vi "ChangeOverGui.vi"() -> ()   [LabVIEW 2016]
uses:
  ChangeOverGui.Properties.ctl
  Logger/Logger.Variant.Sets.ctl
  Station/Station.Changeover.State.vi
  Station/Station.Plate.Properties.ctl
  Sequence/Sequence.Code.SerialFormat.ctl
  Drivers/V7310/LowLevel/V7310.Job.Sets.ctl
  ChangeOverGui.Action.ctl
  Station/Station.State.ctl
  Sequence/Sequence.MainMode.ctl
  Sequence/Sequence.PlateType.ctl
  <vilib>/Utility/miscctls.llb/LVBoundsTypeDef.ctl
  <vilib>/Utility/miscctls.llb/LVRowAndColumnUnsignedTypeDef.ctl
  tools/CitTemplate/citTemplate.errData.ctl
  tools/EventLog/EventLog.EventSource.ctl
  tools/Translator/Translator.Message.ctl
  tools/Config/Config.Global.vi
  Global/ApplicationGlobal.vi
  Station/Station.Global.vi
  Sequence/Sequence.Global.vi
  Drivers/V7310/LowLevel/V7310.Global.vi
  tools/Picture/Rotate.llb/rotate 24bit.vi
panel:
  out "Progress":bool
  out "TotalCounter":u32 caption="Total Counter"
  in  "ShowOrdersTable":bool
  in  "OrdersTable":i32(listbox) caption="Last A"
  in  "ShowPropertiesClient":bool
  out "DoubleOrder":bool
  in  "ShowPropertiesWabco":bool
  in  "Properties":T1={"LaserJob"=0, "AddTxt"="", "FactoryCode"="", "RevID"=0, "ForkID"=0, "Failures Limit"=0, "GlobalCounter"=0, "Bank"=enum."A/B-1", "SerialFormat"=enum."6 dig", "CodeA"={"X"=0.0, "Y"=0.0, "Angle"=0.0}, "CodeB"={"X"=0.0, "Y"=0.0, "Angle"=0.0}, "SetupDMC"=FALSE, "CVX Program"=0} {"CodeB"."Angle" format="%.1f"; "CodeB"."Y" format="%.2f"; "CodeB"."X" format="%.2f"; "CodeA"."Angle" format="%.1f"; "CodeA"."Y" format="%.2f"; "CodeA"."X" format="%.2f"; "LaserJob" items=["", "000 000 000 0", "899 010 203 4", "899 010 206 4", "899 050 124 4", "899 050 145 4", "899 050 146 4", "899 050 146 4v bst3", "899 050 147 4", "899 052 580 4", "899 052 580 4v2", "899 052 582 4", "899 052 930 4", "899 052 942 4", "899 052 942 4 v2", "899 053 089 4", "899 053 089 4v 9325100100", "899 053 096 4", "899 053 096 4 v2", "899 053 502 4", "899 053 522 4", "899 053 524 4", "899 053 527 4", "899 053 803 4 v1", "899 053 803 4 v2", "899 053 803 4 v3", "899 053 803 4 v5 cb1", "899 053 804 4", "899 053 804 4 V2", "899 053 804 4 v 4324101170", "899 053 804 4 v daiml", "899 053 804 4_scania", "899 053 804 4v daimler", "899 053 804 4v daimler2", "899 053 804 4v047", "899 053 814 4", "899 053 814 4 v1", "899 053 814 4_KESKA", "899 053 814 4v sc", "899 053 815 4 ", "899 053 913 4", "899 053 913 4 test", "899 053 913 4 v2", "899 053 923 4", "8990501244", "Karol 899 053 089 4", "VJ Test", "inne"]}
  in  "ViewMode":enum16{"-", "Wabco", "Client"}(ring)
  in  "Serial":T2
  in  "Wabco":cluster{"ProductNo":string, "PlateNo":string}
  in  "Client":cluster{"ProductNo":string, "PlateNo":string}
  out "ClientPlate":picture
  out "Image":picture
  out "WabcoPlate":picture
  out "_loop":i32(ring)=4
  out "Panel":refnum<vi>
  in  "StartHere...":bool
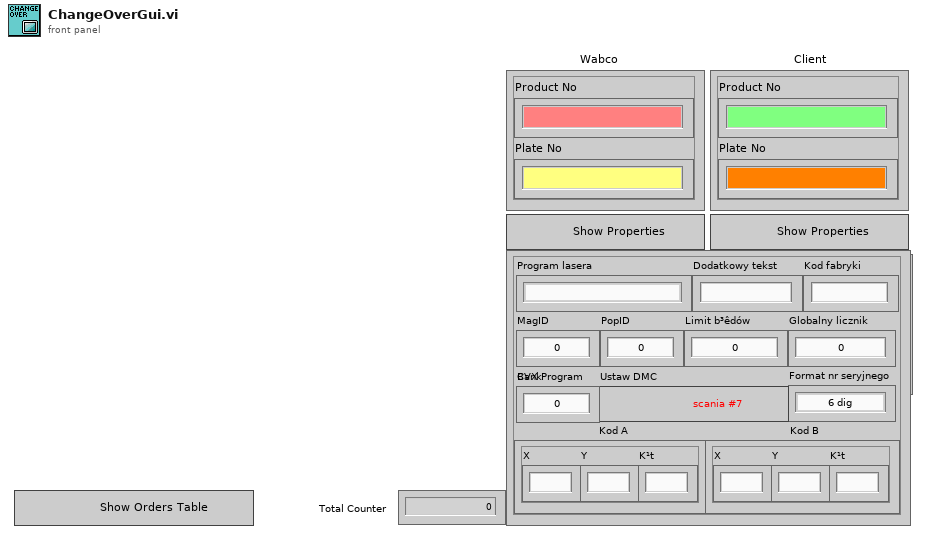
[diagram p1: front panel]
types:
  T1 = typedef "ChangeOverGui.Properties.ctl" = cluster{"LaserJob":u16, "AddTxt":string, "FactoryCode":string, "RevID":u8, "ForkID":u8, "Failures Limit":u16, "GlobalCounter":i32, "Bank":enum8{"A/B-1", "A/B-2", "A/B-3"}, "SerialFormat":enum16{"", "6 dig", "7 dig"}, "CodeA":cluster{"X":dbl, "Y":dbl, "Angle":dbl}, "CodeB":cluster{"X":dbl, "Y":dbl, "Angle":dbl}, "SetupDMC":bool, "CVX Program":u8}
  T2 = cluster{"TotalQuantity":u16, "OrderQuantity":u16, "SerialNo":i32}
  T3 = typedef "Logger.Variant.Sets.ctl" = cluster{"State":T4, "ImgPath":path, "WabcoPlate":string, "WabcoProduct":string, "ClientProduct":string, "ClientPlate":string, "TotalQuantity":u16, "OrderQuantity":u16, "Serial":i32, "Wabco":T5, "Client":T5}
  T4 = typedef "Station.Changeover.State.vi" = enum16{"Init", "Scaning", "NOK", "Wait for ack", "Ready"}
  T5 = typedef "Station.Plate.Properties.ctl" = cluster{"LaserJob":string, "AdditionalTxt":string, "FactoryCode":string, "RevID":u8, "ForkID":u8, "FailuresLimit":u16, "GlobalCnt":i32, "ScannerProgram":u8, "SerialFormat":T6, "CoordA":T7, "CoordB":T7, "DMCconfig":i32, "CVX_Program":u16}
  T6 = typedef "Sequence.Code.SerialFormat.ctl" = enum8{"", "6 dig", "7 dig"}
  T7 = typedef "V7310.Job.Sets.ctl" = cluster{"X":dbl, "Y":dbl, "Angle":dbl}
  T8 = typedef "Station.State.ctl" = enum16{"Idle", "Ready", "Run", "Stop", "Error", "Home", "Done", "Emg"}
  T9 = typedef "ChangeOverGui.Action.ctl" = enum32{"idle", "constructor", "destructor", "---ChangeOverGui ---", "Clear", "Validate", "Read File", "Read Imgs", "Check", "Accept", "Reject", "Scan.Begin", "Scan", "Update Table", "Update Counter", "DMC Accept"}
  T10 = typedef "Sequence.MainMode.ctl" = enum16{"Process", "Base", "Order", "Manual", "Logs", "Results", "Stats", "DMC Config"}
  T11 = typedef "Sequence.PlateType.ctl" = enum16{"Wabco", "Client"}
  T12 = typedef "LVRowAndColumnUnsignedTypeDef.ctl" = cluster{"Row":u32, "Column":u32}
  T13 = typedef "citTemplate.errData.ctl" = cluster{"ts":timestamp, "src":T14, "instance":i32, "action":string, "error":errorcluster, "unconfirmed":bool}
  T14 = typedef "EventLog.EventSource.ctl" = enum16{"All", "Gui", "Ref", "File", "Arch", "Seq", "CPX", "DB", "Laser", "Scan.P", "Scan.O"}
  T15 = enum8{"Enabled", "Disabled", "Disabled and Grayed Out"}
  T16 = typedef "Translator.Message.ctl" = enum16{"-", "Event confirmed", "Log out", "Log in", "Shutdown", "Cancel", "Start", "Begin time", "End time", "Duration", "Service Mode", "Ignore Results", "Serial Format", "On", "Off", "OK", "NOK", "NOK %s", "Home", "Work", "Close", "Open", "In progress...", "Missing", "Empty", "Hardware failure", "Initial", "Default", "Total", "Out of range", "Free disk space is below 1GB - contact technician", "Error %d >> %s", "Error %d >> %s >> %s", "Msg %d >> %s", "Laser msg %d %s", "Laser cmd error %s %d", "Laser cmd failed %s", "Laser cmd warning %s", "Laser disconnected", "Laser status %s", "Laser already started", "Laser job unkonwn %s", "Laser job missing %s", "Laser job select failure %s", "Unable to start laser printing (%s)", "Unable to stop laser printing (%s)", "Laser marking aborted", "Laser marking timeout", "Unable to reset Laser Interlock (%s)", "Unable to trigger Laser. Laser not ready (%s)", "Laser job '%s' coordinates not configured", "Starting %s", "Quitting %s", "Configured", "Initializing", "Quitting", "Loading", "Loaded %d results", "Loaded %d events", "Running", "Stopped", "Summary", "Laser", "Do you want to continue?", "Do you want to delete the configuration?", "The configuration is being used by an order. Unable to delete!", "Press confirm button", "Station is not based. Do you want to exit?", "Station requires changeover. Do you want to run the test?", "Test options are not set as default. Do you want to continue?", "Formatting of WabcoNo is disabled. Do you want to continue?", "Product not detected. Do you want to continue?", "Product scan failed. Do you want to continue?", "Calibration", "Log out?", "System", "All", "IDLE", "Translating...%s", "Not found", "Alarm %s", "Run", "Skip", "Abort", "Repeat", "Please wait...", "Database disconnected", "Database disconnected - changeover disabled!", "Login to database successful", "Login to database failed: %d; %s", "Unable to check the product status of reference %d - database disconnected", "Unable to set the product status of reference %d - database disconnected", "Variant file backup %s", "Read variant (%s)", "Result", "Station armed!", "Station requires changeover!", "Select reference number...", "EMERGENCY BUTTON - press Control button", "EMERGENCY DOOR - press Control button", "Resetting Emergency...", "Unable to reset safety circuit - Emergency Button pressed", "Unable to reset safety circuit - Emergency Side Door open", "Station not based", "Station based", "Station not empty", "Station basing...", "No order", "Press Start to begin new order", "Scanning new order", "Order NOK. Correct or scan again", "Order OK. Press Accept", "Order ready", "Revolver incorrect", "Fork incorrect", "Revolver missing", "Revolver empty", "Container missing", "Offline results", "Offline statistics", "Updating statistics %.1f %%", "DMC Configurator", "Door open", "Close the front door", "Press start button", "Done. Open the front door", "Running...", "Running...%.1f %%", "Pause %s", "Pause %s. NOK container missing", "Pause %s. OK container missing", "Pause %s. Revolver empty", "Pause %s. Revolver missing", "Pause %s. Revolver incorrect", "Pause %s. Fork missing", "Pause %s. Fork incorrect", "Pause %s. Too many failures", "Pause %s. Unloading failure", "Pause %s. One slot is not working", "Pause %s. Part order is done. Empty OK container", "Pause %s. Unable to move product to slot", "Pause %s. Unable to move back product pusher", "Pause %s. Unable to lift product", "Pause %s. Unable to move back product lifter", "Pause %s. Unable to move product arm to Work", "Pause %s. Unable to move product arm to NOK", "Pause %s. Unable to move product arm to OK", "Pause %s. Unable to unsuck the NOK product", "Pause %s. Unable to drop the NOK product", "Pause %s. Product OK missing", "Pause %s. Unable to unsuck the OK product", "Pause %s. Unable to drop the OK product", "Stopping...", "File '%s' is missing", "File '%s' is broken", "File '%s' is running", "Log file started (%s)", "Log file ended (%s)", "Log file stopped (%s)", "Log file ignored (%s)", "Log file exported (%s)", "Log file export failed (%s)", "Wrong serial number in log file", "Wrong reference number in log file", "Test steps are missing", "%s = %.3f", "Process param '%s' not found in DB", "Process param '%s' wrong order", "Process param '%s' value %.3f out of limits (%.3f; %.3f)", "Step%d param '%s' not found in DB", "Step%d param '%s' wrong order", "Step%d param '%s' value %.3f out of limits (%.3f; %.3f)", "Step%d EV '%s' not found in DB", "Step%d EV '%s' wrong order", "\"%s\" not found in DB", "\"%s\" wrong order", "\"%s\" value %.3f out of limits (%.3f; %.3f)", "\"%s\" not found in software", "Process init (%s)", "Process started", "Process restarted", "Process run", "Process done", "Process done - remove OK container", "Process aborted", "Process aborted at work", "Process aborted at home", "Process error", "Process error at home", "Process error at work", "Process close", "Process pause", "Process continue", "Process door open", "Process door close", "Process pause at slot %s due to %s", "Select plate from the order to process", "Do you want to start the process?", "Do you want to continue the process?", "There is unfinished order. Do you want to put the new order?", "Product %s %d OK", "Product %s %d NOK", "Unable to unload the slot %s. Product missing in the slot", "Unable to unload the slot %s. Product already in the arm", "Unable to accept the product as OK. Product missing in slot %s", "Unable to accept the product as OK. Product could not drop into the container at slot %s", "Unable to accept the product as NOK. Product could not drop into the container at slot %s", "Scan failed. Error %s", "Scan failed. Scanner disconnected", "Scan failed. Wrong Wabco number %d, limit (%d,%d)", "Scan failed. Wrong serial number %d, limit (%d,%d)", "Scan failed. Wrong date %d, limit (%d,%d)", "Scan failed. Wrong product wabco number %d (expected %d)", "Scan failed. Wrong product serial number %d (expected > 0)", "Scan OK %s", "Scan failed. Unable to determine table position (%s)", "Scan failed. Timeout", "Tune failed. Scanner disconnected", "Tune failed. Timeout", "%s = %d", "%s = %d->%d", "Unable to set %s = %.2f - Air Pressure Inside off", "Unable to set digital output '%s' = %d", "Unable to activate air pressure inside - timeout", "Unable to activate air pressure inside - aborted", "Unable to switch on Air Main Valve - Air Pressure Inlet off", "Unable to switch on Air Main Valve - Door open", "Unable to switch off Air Main Valve - timeout", "Unable to switch off Air Main Valve - aborted", "Unable to rotate Table - timeout", "Unable to rotate Table - aborted", "Unable to rotate Table - Product Move not in Home position", "Unable to rotate Table - Air Pressure Inside off", "Unable to rotate Table - Product Lift A not in Home position", "Unable to rotate Table - Product Lift B not in Home position", "Unable to rotate Table - unlock before movement timeout", "Unable to rotate Table - lock after movement timeout", "Unable to move Table Lock to %s position - timeout", "Unable to move Table Lock to %s position - aborted", "Unable to move Table Lock to %s position - Air Pressure Inside off", "Unable to move Table Lock to %s position - Table not in position", "Unable to move Product Lift A to %s position - timeout", "Unable to move Product Lift B to %s position - timeout", "Unable to move Product Lift A to %s position - aborted", "Unable to move Product Lift B to %s position - aborted", "Unable to move Product Lift A to %s position - Air Pressure Inside off", "Unable to move Product Lift B to %s position - Air Pressure Inside off", "Unable to move Product Lift A to %s position - Table not locked", "Unable to move Product Lift B to %s position - Table not locked", "Unable to move Product Lift A to %s position - Product Arm not in Work position", "Unable to move Product Lift B to %s position - Product Arm not in Work position", "Unable to set Product Suction Gripper %s to %s - timeout", "Unable to set Product Suction Gripper %s to %s - aborted", "Unable to set Product Suction Gripper %s to %s - Air Pressure Inside off", "Unable to set Product Suction Gripper %s to %s - Table slot unkown", "Unable to move Product Arm to %s position - timeout", "Unable to move Product Arm to %s position - aborted", "Unable to move Product Arm to %s position - Air Pressure Inside off", "Unable to move Product Arm to %s position - Product Lift A not in Home position", "Unable to move Product Arm to %s position - Product Lift B not in Home position", "Unable to move Product to %s position - timeout", "Unable to move Product to %s position - aborted", "Unable to move Product to %s position - Air Pressure Inside off", "Unable to move Product to %s position - Table not in position"}
  T17 = typedef "citTemplate.notifierHandle.ctl" = refnum<notifier>
  T18 = enum32{"Invalid", "Standard", "Closed", "Hidden", "Minimized", "Maximized"}
  T19 = typedef "Station.Data.ctl" = cluster{"State":T8, "Seq.State":T20, "Seq.BreakReason":T21, "Seq.BreakSource":T22, "Hw failure":bool, "Unconfirmed":bool, "Station empty":bool, "Home err":bool, "Order done":bool, "DUT present":T23, "EmgState":T24, "Sets":T25, "StatusBits":T27}
  T20 = typedef "Sequence.State.ctl" = enum16{"Init", "Idle", "Home", "Work", "Run", "Pause"}
  T21 = typedef "Sequence.Test.BreakReason.ctl" = enum16{"-", "NOK container", "OK container", "Rev empty", "Rev missing", "Rev wrong", "Fork missing", "Fork wrong", "NOK limit", "Unload failure", "Single slot", "Part done", "Err: Prod move work", "Err: Prod move home", "Err: Prod lift work", "Err: Prod lift home", "Err: Prod Arm Work", "Err: Prod Arm NOK", "Err: Prod Arm OK", "Err: Prod NOK suck", "Err: Prod NOK drop", "Err: Prod OK missing", "Err: Prod OK suck", "Err: Prod OK drop"}
  T22 = typedef "Sequence.Test.BreakSource.ctl" = enum16{"-", "A", "B", "A/B"}
  T23 = typedef "FestoCPX.Station.ProdPresent.ctl" = cluster{"Slot1":cluster{"A":bool, "B":bool}, "Slot2":cluster{"A":bool, "B":bool}, "Slot3":cluster{"A":bool, "B":bool}, "Slot4":cluster{"A":bool, "B":bool}, "Final":cluster{"A":bool, "B":bool}, "OK":cluster{"A":bool, "B":bool}, "Container":cluster{"OK":bool, "NOK":bool}}
  T24 = typedef "FestoCPX.Station.EmgState.ctl" = cluster{"Button":bool, "SideDoor":bool, "FrontDoor":bool, "DoorSecured":bool}
  T25 = typedef "Sequence.UserData.ctl" = cluster{"GuiMode":T10, "Test":T26, "ContinueOrder":bool}
  T26 = typedef "MainGui.TestOptions.ctl" = cluster{"IgnoreResults":bool, "IgnoreImages":bool, "ServiceMode":bool}
  T27 = typedef "Station.Home.Status.Bits.ctl" = cluster{"Door Close":bool, "Rev OK":bool, "Fork OK":bool, "Container OK":bool, "Station empty":bool}
  T28 = typedef "LVBoundsTypeDef.ctl" = cluster{"Width":u32, "Height":u32}
  T29 = typedef "LVPositionTypeDef.ctl" = cluster{"Left":i32, "Top":i32}
  T30 = typedef "Sequence.Data.ctl" = cluster{"BeginTS":timestamp, "EndTS":timestamp, "State":T20, "Status.Work":T31, "Status.Process":T31, "Status.Home":T31, "Status.Wabco":T31, "Status.Client":T31, "BreakReason":T21, "BreakSource":T22, "DoorLock":bool, "Status.Prod":T32[], "UserAction":T36, "UserData":T25, "Error":errorcluster, "Code":T37, "Rotations":i32, "ProdIdx":i32, "ProdDone":T32[], "PrintedSerials-Wabco":i32[], "PrintedSerials-Client":i32[], "Counters-Wabco":T38, "Counters-Client":T38}
  T31 = typedef "Sequence.Step.Status.ctl" = enum16{"-", "Pending", "Running", "Skipped", "Passed", "Failed", "Done", "Error", "Aborted", "Stopped"}
  T32 = typedef "Sequence.Test.Status.ctl" = cluster{"Slot":T33, "A":T35, "B":T35}
  T33 = typedef "Sequence.Slot.StatusData.ctl" = cluster{"ID":i32, "Unload":T34, "TS":timestamp, "duration":u32}
  T34 = typedef "Sequence.Test.Unload.Status.ctl" = enum16{"init", "check NOK", "check OK", "wait on NOK", "wait on OK", "wait on Unload", "done"}
  T35 = typedef "Sequence.Prod.StatusData.ctl" = cluster{"status":T31, "pause":T21, "present":bool, "printed":bool, "scanned":bool, "tuned":bool, "removed":bool, "OCRignored":bool, "LaserVariables":string[], "Serial":i32, "path":path, "corners":cluster{"X":i32, "Y":i32}[], "verification":u8, "ScanerReadOut":string[]}
  T36 = typedef "Sequence.UserActions.ctl" = cluster{"Stop":bool, "Pause":bool, "Next":bool}
  T37 = typedef "Sequence.Code.Sets.ctl" = cluster{"Ready":bool, "DoubleOrder":bool, "OrderDone":bool, "AllowSingleSlot":bool, "IgnoreOCR":bool, "ThresholdA":u8, "ThresholdB":u8, "Plate":T11, "ImgPath":path, "Variant":T3}
  T38 = typedef "Sequence.Counters.ctl" = cluster{"Expected":u16, "Done":u16, "OK":u16, "NOK":u16, "NOKlimit":u16, "Part":u16, "PartOK":u16}
  T39 = typedef "V7310.Data.Status.ctl" = cluster{"State":T40, "LaserStatus":T41, "LaserStatusRaw":string, "Ref":refnum<k5>, "RTC TS":timestamp, "Conn TS":timestamp, "Msg":T42[], "JobInUse":string, "Jobs":string[], "Vars":T43[]}
  T40 = typedef "V7310.Data.Status.State.ctl" = enum16{"First", "Init", "Msg", "Error", "Abort", "Idle", "Run"}
  T41 = typedef "V7310.LaserStatus.ctl" = enum16{"-", "FatalError", "Initialize", "KeySwitchOpen", "TimeoutInterlock", "InterlockOpen", "StartUp", "ShutterlockOpen", "Standby", "Ready", "PrepareForMarking", "WaitForTrigger", "Marking"}
  T42 = typedef "V7310.Message.Data.ctl" = cluster{"ID":i32, "Msg":string}
  T43 = typedef "V7310.Job.Variable.ctl" = cluster{"Name":string, "Value":string}
  T44 = typedef "DMCConfiguatorGui.ConfigData.ctl" = cluster{"CreateDate":timestamp, "Name":string, "Components":T45[]}
  T45 = typedef "DMCConfiguatorGui.Component.ctl" = cluster{"Type":T46, "Var":T47, "Text":string}
  T46 = typedef "DMCConfiguatorGui.Type.ctl" = enum8{"Text", "Variable"}
  T47 = typedef "DMCConfiguatorGui.Var.ctl" = enum8{"-", "Wabco No", "Client No", "Serial", "Date"}
  T48 = typedef "imagedata.ctl" = cluster{"image type":i32, "image depth":i32, "image":u8[], "mask":u8[], "colors":u32[], "Rectangle":cluster{"left":i16, "top":i16, "right":i16, "bottom":i16}}
  T49 = cluster{"WabcoProduct":string, "WabcoPlate":string}
  T50 = cluster{"ClientProduct":string, "ClientPlate":string}
  T51 = cluster{"TotalQuantity":u16, "OrderQuantity":u16, "Serial":i32}
  T52 = typedef "Keyence.CodeDetails.ctl" = cluster{"text":string, "status":bool, "corners":cluster{"X":i32, "Y":i32}[], "level":u8, "class":string, "path":path}
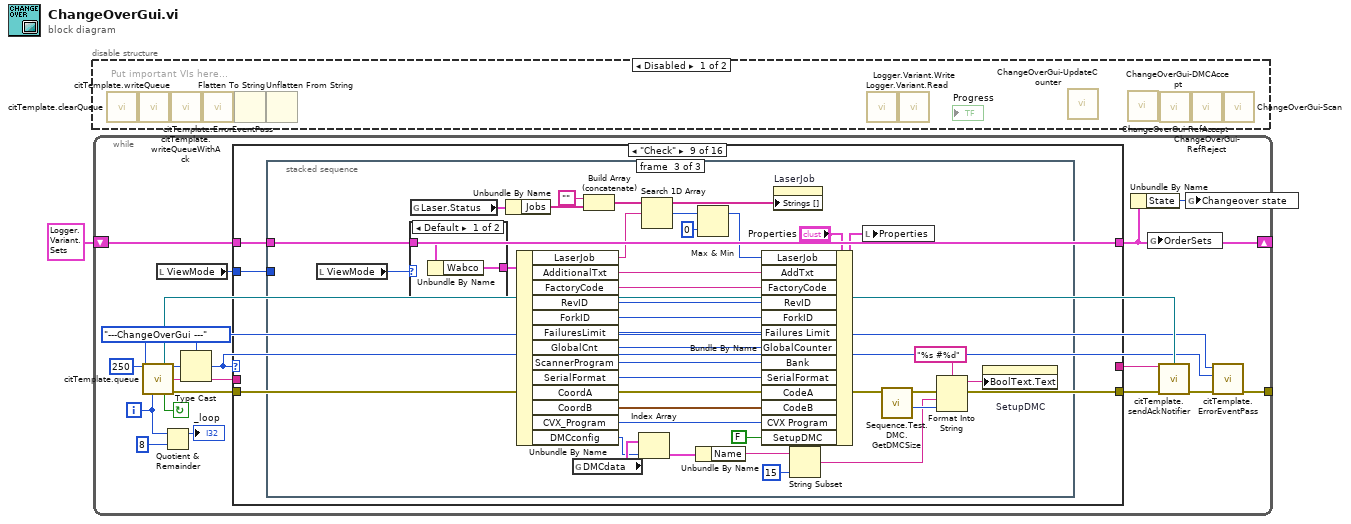
[diagram p0: block diagram]
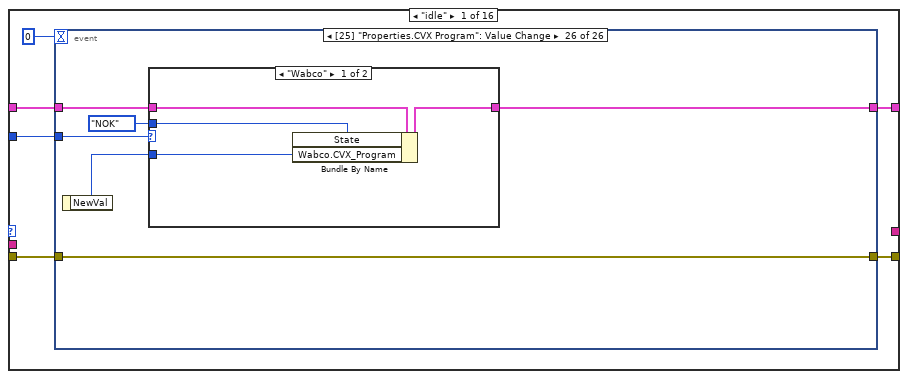
[diagram p3: hidden frame]
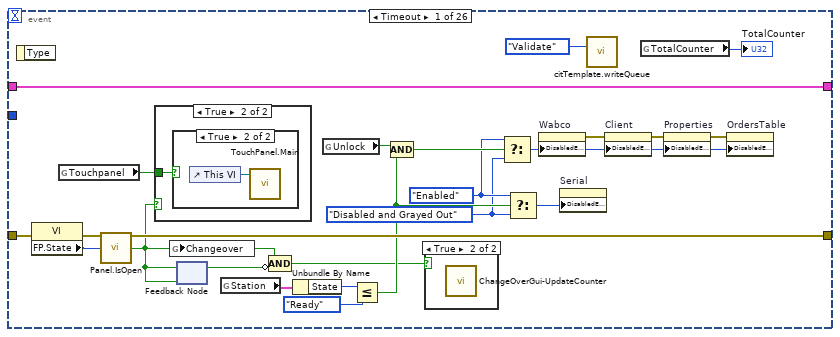
[diagram p4: hidden frame]
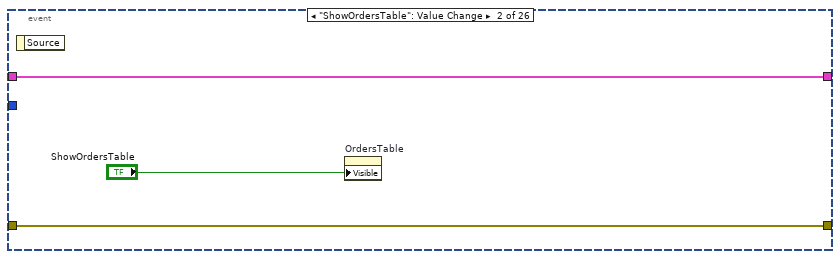
[diagram p8: hidden frame]
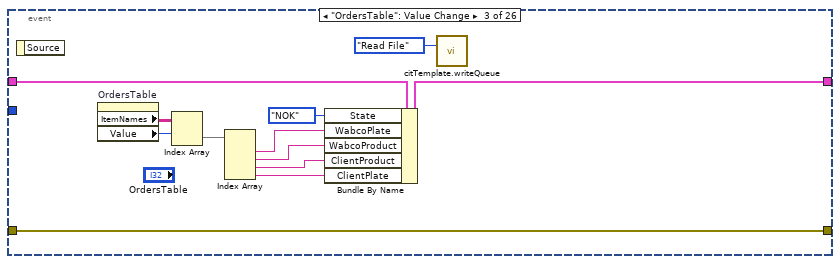
[diagram p9: hidden frame]
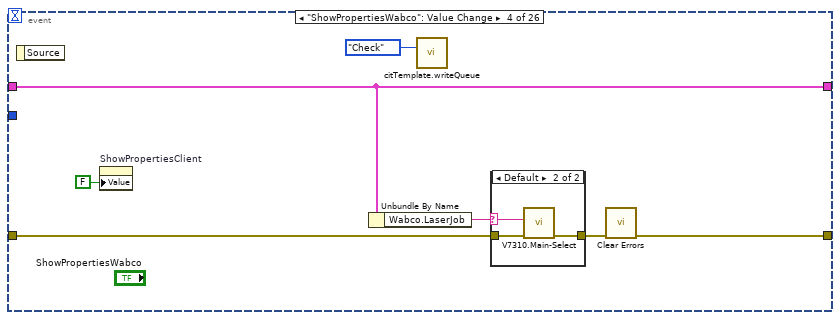
[diagram p10: hidden frame]
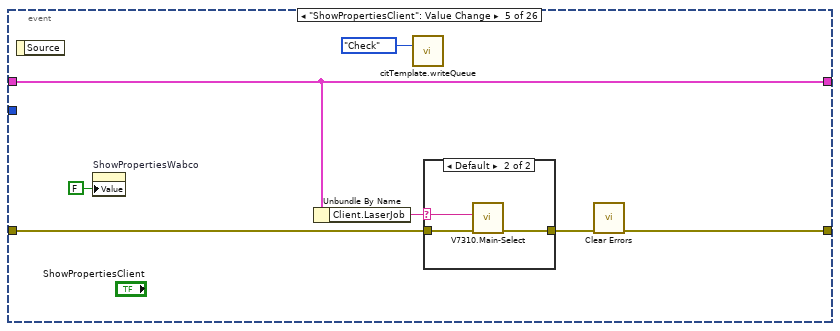
[diagram p12: hidden frame]
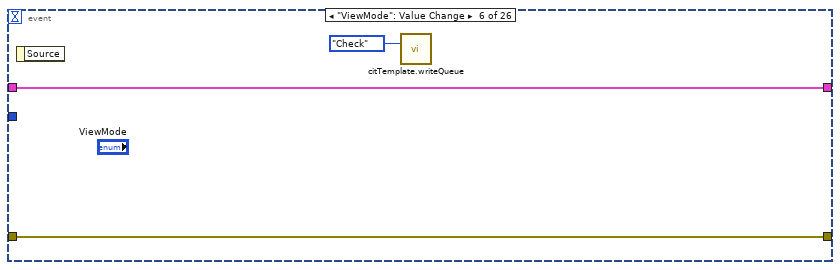
[diagram p14: hidden frame]
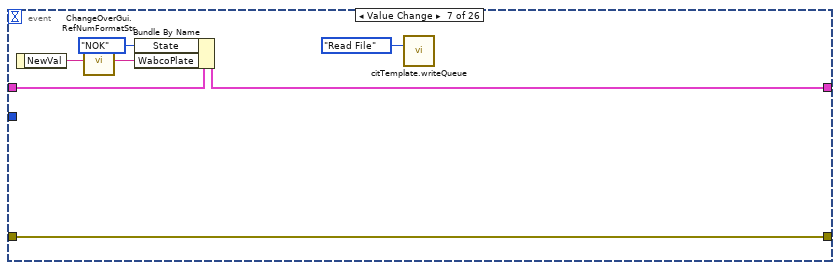
[diagram p15: hidden frame]
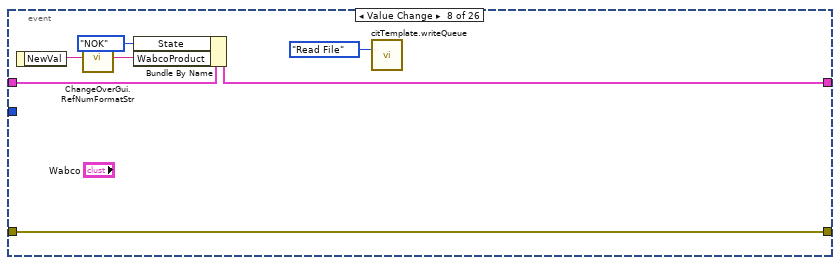
[diagram p16: hidden frame]
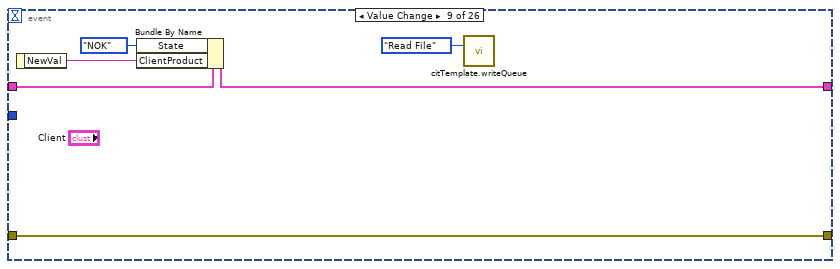
[diagram p17: hidden frame]
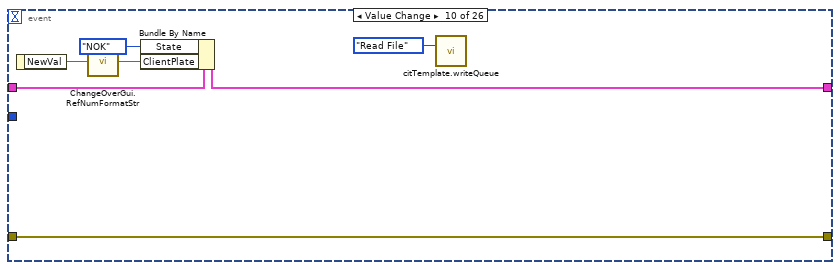
[diagram p18: hidden frame]
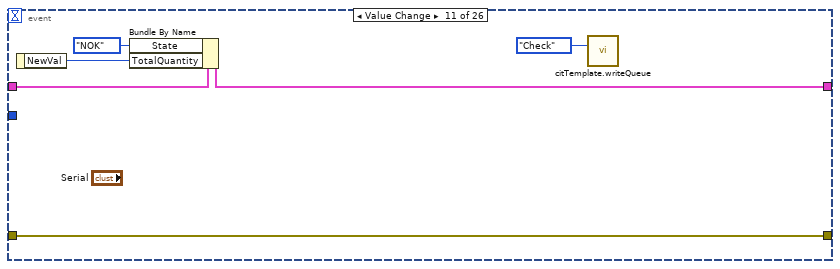
[diagram p19: hidden frame]
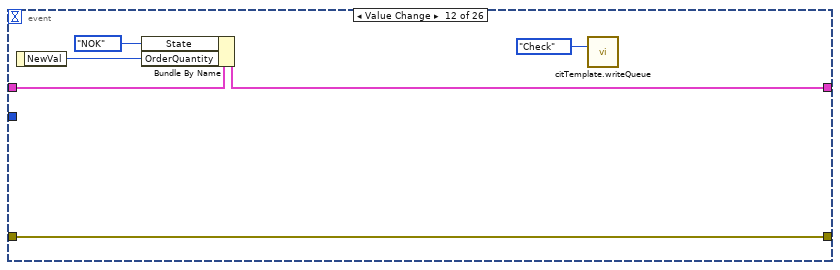
[diagram p20: hidden frame]
diagram:
  n1 = disable-structure shown="Disabled" {
    frame Disabled {
      # "Put important VIs here..."
      n2 = call "citTemplate.clearQueue.vi"() -> ()  [unwired: 14 in, 2 out]
      n3 = call "citTemplate.writeQueue.vi"() -> ()  [unwired: 15 in, 1 out]
      n4 = call "citTemplate.writeQueueWithAck.vi"() -> ()  [unwired: 13 in, 3 out]
      n5 = call "citTemplate.ErrorEventPass.vi"() -> ()  [unwired: 11 in, 1 out]
      n6 = Flatten To String() -> ()  [unwired: 4 in, 3 out]
      n7 = Unflatten From String() -> ()  [unwired: 5 in, 3 out]
      n8 = call "Logger.Variant.Read.vi"() -> ()  [unwired: 6 in, 6 out]
      n9 = call "Logger.Variant.Write.vi"() -> ()  [unwired: 11 in, 1 out]
      n10 = call "ChangeOverGui-UpdateCounter.vi"() -> ()  [unwired: 11 in, 1 out]
      n11 = call "ChangeOverGui-DMCAccept.vi"() -> ()  [unwired: 11 in, 1 out]
      n12 = call "ChangeOverGui-RefAccept.vi"() -> ()  [unwired: 11 in, 1 out]
      n13 = call "ChangeOverGui-RefReject.vi"() -> ()  [unwired: 11 in, 1 out]
      n14 = call "ChangeOverGui-Scan.vi"() -> ()  [unwired: 11 in, 1 out]
    }
    frame Enabled {
    }
  }
  n15 = while {
    tunnel: [w7] -> _
    shift-right: [w2] -> _
    shift-left: T3 {"State"=enum."Init", "ImgPath"=path "", "WabcoPlate"="", "WabcoProduct"="", "ClientProduct"="", "ClientPlate"="", "TotalQuantity"=0, "OrderQuantity"=0, "Serial"=0, "Wabco"={"LaserJob"="", "AdditionalTxt"="037", "FactoryCode"="", "RevID"=0, "ForkID"=0, "FailuresLimit"=0, "GlobalCnt"=0, "ScannerProgram"=0, "SerialFormat"=enum."6 dig", "CoordA"={"X"=0.0, "Y"=0.0, "Angle"=0.0}, "CoordB"={"X"=0.0, "Y"=0.0, "Angle"=0.0}, "DMCconfig"=0, "CVX_Program"=0}, "Client"={"LaserJob"="", "AdditionalTxt"="", "FactoryCode"="037", "RevID"=0, "ForkID"=0, "FailuresLimit"=0, "GlobalCnt"=0, "ScannerProgram"=0, "SerialFormat"=enum."6 dig", "CoordA"={"X"=0.0, "Y"=0.0, "Angle"=0.0}, "CoordB"={"X"=0.0, "Y"=0.0, "Angle"=0.0}, "DMCconfig"=0, "CVX_Program"=0}} ("VariantSets out") -> [w5]
    i -> [w9]
    stop <- w16 continue-if-true
    w13 = ChangeOverGui.Action."---ChangeOverGui ---" ("Action")
    n16 = call "citTemplate.queue.vi"("ms timeout (250 ms)"=250, "event enum"=w13, "iteration (-1)"=w9) -> ("notifierHandle out"=w15:T17, "event out"=w19:u32, "(flatten) data out"=w18:string, "continue"=w16:bool, "error out"=w17:errorcluster)  [unwired: 2 in, 6 out]
    n17 = local read "ViewMode"() -> (w3:enum16{"-", "Wabco", "Client"})
    n18 = Quotient & Remainder(x=w9, y=8) -> (x-y*floor(x/y)=→"_loop":i32)  [unwired: 1 out]
    n19 = Type Cast(type=w13, x=w19) -> (*(type *) &x=w8:T9)
    n20 = case shown="\"Check\"" w8 {
      tunnel: w18 -> [_ _ _ w388 _ _ _ _ _ _ _ _ _ _ _ w1045]
      tunnel: w17 -> [w24 w334 w378 w387 w420 w428 w691 w694 w748 w825 w842 w855 w863 w1001 w1030 w1044]
      tunnel: [_ _ _ "" _ _ _ _ _ _ _ _ _ _ _ ""] -> w14
      tunnel: [w23 w333 w377 w381 w420 w428 w688 w694 w748 w824 w841 w855 w859 w1001 w1030 w1038] -> w12
      tunnel: [w21 w331 w372 w380 w421 w425 w689 w693 w747 w822 w837 w851 w865 w1002 w1029 w1037] -> w2
      tunnel: w5 -> [w22 w332 w372 w380 w421 w426 w690 w693 w747 w823 _ _ w866 w1002 w1029 w1042]
      tunnel: w3 -> [w20 _ _ _ _ w423 _ _ w746 _ _ _ _ _ w1021 w1036]
      frame "idle" {
        n21 = event shown="[25] \"Properties.CVX Program\": Value Change" {
          selector: _ -> [_ _ _ _ _ _ _ _ _ _ _ _ _ _ _ _ _ _ _ _ _ _ _ _ _ _]
          dyn-events: _ -> [_ _ _ _ _ _ _ _ _ _ _ _ _ _ _ _ _ _ _ _ _ _ _ _ _ _]
          timeout: 0 -> [_ _ _ _ _ _ _ _ _ _ _ _ _ _ _ _ _ _ _ _ _ _ _ _ _ _]
          tunnel: w24 -> [w48 w53 w65 w69 w80 w90 w95 w101 w108 w117 w123 w129 w135 w144 w161 w176 w191 w206 w221 w236 w251 w266 w281 w296 w312 w322]
          tunnel: [w46 w53 w65 w66 w77 w90 w95 w101 w108 w117 w123 w129 w135 w144 w161 w176 w191 w206 w221 w236 w251 w266 w281 w296 w314 w322] -> w23
          tunnel: w22 -> [w44 w52 w62 w70 w81 w89 w97 w104 w110 w116 w122 w128 w134 w140 w160 w174 w189 w204 w218 w233 w248 w263 w278 w293 w310 w321]
          tunnel: [w44 w52 w61 w70 w81 w89 w94 w102 w106 w115 w121 w127 w133 w139 w159 w173 w188 w203 w217 w232 w246 w262 w275 w290 w310 w317] -> w21
          tunnel: w20 -> [_ _ _ _ _ _ _ _ _ _ _ _ _ w137 w155 w172 w187 w202 w216 w230 w247 w260 w277 w292 w305 w320]
          event Timeout {
            w31 = T15."Disabled and Grayed Out" ("Disabled")
            w32 = T15."Enabled" ("Disabled")
            n22 = event-data() -> ()  [unwired: 2 out]
            n23 = property class="VI"(error in=w48) -> (error out=w46:errorcluster, "FP.State"=w43:T18)  [unwired: 1 in, 1 out]
            n24 = global read "Config.Global.vi" "Touchpanel"() -> (w47:bool)
            n25 = call "Panel.IsOpen.vi"("FP State"=w43) -> ("Open?"=w26:bool)
            n26 = case shown="True" w26 {
              tunnel: w47 -> [_ w49]
              frame False {
              }
              frame True {
                n27 = case shown="True" w49 {
                  frame False {
                  }
                  frame True {
                    n28 = control-ref of="This VI"() -> (w50:refnum<vi>)
                    n29 = call "TouchPanel.Main.vi"("VI ref"=w50) -> ()  [unwired: 8 in, 3 out]
                  }
                }
              }
            }
            n30 = global write "Station.Global.vi" "Changeover"(w26) -> ()
            n31 = feedback-in #1(w26) -> ()
            n32 = feedback #1(w26) -> (w30:bool)
            n33 = global read "Station.Global.vi" "Station"() -> (w39:T19)
            n34 = Compound Arithmetic op=AND(w26, invert w30) -> (w28:bool)
            n35 = Unbundle By Name(w39) -> ("State"=w29:T8)
            n36 = global read "ApplicationGlobal.vi" "Unlock"() -> (w41:bool)
            n37 = Less Or Equal?(x=w29, y=Station.State."Ready") -> (x <= y?=w33:bool)
            n38 = Compound Arithmetic op=AND(w41, w33) -> (w34:bool)
            n39 = case shown="True" w28 {
              frame False {
              }
              frame True {
                n40 = call "ChangeOverGui-UpdateCounter.vi"() -> ()  [unwired: 11 in, 1 out]
              }
            }
            n41 = Select(t=w32, s=w34, f=w31) -> (s? t:f=w35:T15)
            n42 = Select(t=w32, s=w33, f=w31) -> (s? t:f=w37:T15)
            n43 = property on="Wabco" class="Clust (strict)"("DisabledEnum"=w35) -> (error out=w42:errorcluster)  [unwired: 2 in, 1 out]
            n44 = property on="Serial" class="Clust (strict)"("DisabledEnum"=w37) -> ()  [unwired: 2 in, 2 out]
            n45 = call "citTemplate.writeQueue.vi"("event in (if not connected:all statemachine with data event)"=ChangeOverGui.Action."Validate" ("Action")) -> ()  [unwired: 14 in, 1 out]
            n46 = property on="Client" class="Clust (strict)"(error in=w42, "DisabledEnum"=w35) -> (error out=w40:errorcluster)  [unwired: 1 in, 1 out]
            n47 = global read "ApplicationGlobal.vi" "TotalCounter"() -> (→"TotalCounter":u32)
            n48 = property on="Properties" class="Clust (strict)"(error in=w40, "DisabledEnum"=w35) -> (error out=w36:errorcluster)  [unwired: 1 in, 1 out]
            n49 = property on="OrdersTable" class="MCListbox (strict)"(error in=w36, "DisabledEnum"=w35) -> ()  [unwired: 1 in, 2 out]
          }
          event "ShowOrdersTable": Value Change {
            n50 = event-data() -> ()  [unwired: 2 out]
            n51 = property on="OrdersTable" class="MCListbox (strict)"("Visible"="ShowOrdersTable") -> ()  [unwired: 2 in, 2 out]
          }
          event "OrdersTable": Value Change {
            n52 = event-data() -> ()  [unwired: 2 out]
            n53 = property on="OrdersTable" class="MCListbox (strict)"() -> ("ItemNames"=w63:string[][], "Value"=w64:i32)  [unwired: 2 in, 2 out]
            n54 = Index Array(array=w63, index (row)=w64) -> (element=w60:string[])  [unwired: 1 in]
            n55 = Index Array(array=w60) -> (element #1=w59:string, element #2=w58:string, element #3=w57:string, element #4=w56:string)  [unwired: 4 in]
            n56 = Bundle By Name(cluster=w62, "State"=Station.Changeover.State.vi."NOK", "WabcoPlate"=w59, "WabcoProduct"=w58, "ClientProduct"=w57, "ClientPlate"=w56) -> (w61:T3)
            n57 = call "citTemplate.writeQueue.vi"("event in (if not connected:all statemachine with data event)"=ChangeOverGui.Action."Read File" ("Action")) -> ()  [unwired: 14 in, 1 out]
          }
          event "ShowPropertiesWabco": Value Change {
            n58 = event-data() -> ()  [unwired: 2 out]
            n59 = property on="ShowPropertiesClient" class="Bool (strict)"("Value"=FALSE ("ShowPropertiesClient")) -> ()  [unwired: 2 in, 2 out]
            n60 = Unbundle By Name(w70) -> ("Wabco.LaserJob"=w67:string)
            n61 = call "citTemplate.writeQueue.vi"("event in (if not connected:all statemachine with data event)"=ChangeOverGui.Action."Check" ("Action")) -> ()  [unwired: 14 in, 1 out]
            n62 = case shown="Default" w67 {
              selector: w67 -> [_ w74]
              tunnel: w69 -> [w73 w76]
              tunnel: [w73 w75] -> w68
              frame "" {
              }
              frame Default {
                n63 = call "V7310.Main-Select.vi"("error in"=w76, "Name"=w74) -> ("error out"=w75:errorcluster)  [unwired: 8 in, 1 out]
              }
            }
            n64 = call <vilib>:"Clear Errors.vi"("error in (no error)"=w68) -> ("error out"=w66:errorcluster)  [unwired: 5 in, 1 out]
          }
          event "ShowPropertiesClient": Value Change {
            n65 = event-data() -> ()  [unwired: 2 out]
            n66 = property on="ShowPropertiesWabco" class="Bool (strict)"("Value"=FALSE ("ShowPropertiesWabco")) -> ()  [unwired: 2 in, 2 out]
            n67 = Unbundle By Name(w81) -> ("Client.LaserJob"=w78:string)
            n68 = call "citTemplate.writeQueue.vi"("event in (if not connected:all statemachine with data event)"=ChangeOverGui.Action."Check" ("Action")) -> ()  [unwired: 14 in, 1 out]
            n69 = case shown="Default" w78 {
              selector: w78 -> [_ w85]
              tunnel: w80 -> [w84 w87]
              tunnel: [w84 w86] -> w79
              frame "" {
              }
              frame Default {
                n70 = call "V7310.Main-Select.vi"("error in"=w87, "Name"=w85) -> ("error out"=w86:errorcluster)  [unwired: 8 in, 1 out]
              }
            }
            n71 = call <vilib>:"Clear Errors.vi"("error in (no error)"=w79) -> ("error out"=w77:errorcluster)  [unwired: 5 in, 1 out]
          }
          event "ViewMode": Value Change {
            n72 = event-data() -> ()  [unwired: 2 out]
            n73 = call "citTemplate.writeQueue.vi"("event in (if not connected:all statemachine with data event)"=ChangeOverGui.Action."Check" ("Action")) -> ()  [unwired: 14 in, 1 out]
          }
          event "Wabco.PlateNo": Value Change {
            n74 = event-data() -> ("NewVal"=w93:string)  [unwired: 1 out]
            n75 = call "ChangeOverGui.RefNumFormatStr.vi"("RefNum in"=w93) -> ("RefNum out"=w92:string)  [unwired: 2 out]
            n76 = Bundle By Name(cluster=w97, "State"=Station.Changeover.State.vi."NOK", "WabcoPlate"=w92) -> (w94:T3)
            n77 = call "citTemplate.writeQueue.vi"("event in (if not connected:all statemachine with data event)"=ChangeOverGui.Action."Read File" ("Action")) -> ()  [unwired: 14 in, 1 out]
          }
          event "Wabco.ProductNo": Value Change {
            n78 = event-data() -> ("NewVal"=w100:string)  [unwired: 1 out]
            n79 = call "ChangeOverGui.RefNumFormatStr.vi"("RefNum in"=w100) -> ("RefNum out"=w99:string)  [unwired: 2 out]
            n80 = Bundle By Name(cluster=w104, "State"=Station.Changeover.State.vi."NOK", "WabcoProduct"=w99) -> (w102:T3)
            n81 = call "citTemplate.writeQueue.vi"("event in (if not connected:all statemachine with data event)"=ChangeOverGui.Action."Read File" ("Action")) -> ()  [unwired: 14 in, 1 out]
          }
          event "Client.ProductNo": Value Change {
            n82 = event-data() -> ("NewVal"=w109:string)  [unwired: 1 out]
            n83 = Bundle By Name(cluster=w110, "State"=Station.Changeover.State.vi."NOK", "ClientProduct"=w109) -> (w106:T3)
            n84 = call "citTemplate.writeQueue.vi"("event in (if not connected:all statemachine with data event)"=ChangeOverGui.Action."Read File" ("Action")) -> ()  [unwired: 14 in, 1 out]
          }
          event "Client.PlateNo": Value Change {
            n85 = event-data() -> ("NewVal"=w114:string)  [unwired: 1 out]
            n86 = call "ChangeOverGui.RefNumFormatStr.vi"("RefNum in"=w114) -> ("RefNum out"=w113:string)  [unwired: 2 out]
            n87 = Bundle By Name(cluster=w116, "State"=Station.Changeover.State.vi."NOK", "ClientPlate"=w113) -> (w115:T3)
            n88 = call "citTemplate.writeQueue.vi"("event in (if not connected:all statemachine with data event)"=ChangeOverGui.Action."Read File" ("Action")) -> ()  [unwired: 14 in, 1 out]
          }
          event "Serial.TotalQuantity": Value Change {
            n89 = event-data() -> ("NewVal"=w119:u16)  [unwired: 1 out]
            n90 = Bundle By Name(cluster=w122, "State"=Station.Changeover.State.vi."NOK", "TotalQuantity"=w119) -> (w121:T3)
            n91 = call "citTemplate.writeQueue.vi"("event in (if not connected:all statemachine with data event)"=ChangeOverGui.Action."Check" ("Action")) -> ()  [unwired: 14 in, 1 out]
          }
          event "Serial.OrderQuantity": Value Change {
            n92 = event-data() -> ("NewVal"=w125:u16)  [unwired: 1 out]
            n93 = Bundle By Name(cluster=w128, "State"=Station.Changeover.State.vi."NOK", "OrderQuantity"=w125) -> (w127:T3)
            n94 = call "citTemplate.writeQueue.vi"("event in (if not connected:all statemachine with data event)"=ChangeOverGui.Action."Check" ("Action")) -> ()  [unwired: 14 in, 1 out]
          }
          event "Serial.SerialNo": Value Change {
            n95 = event-data() -> ("NewVal"=w131:i32)  [unwired: 1 out]
            n96 = Bundle By Name(cluster=w134, "State"=Station.Changeover.State.vi."NOK", "Serial"=w131) -> (w133:T3)
            n97 = call "citTemplate.writeQueue.vi"("event in (if not connected:all statemachine with data event)"=ChangeOverGui.Action."Check" ("Action")) -> ()  [unwired: 14 in, 1 out]
          }
          event Value Change {
            n98 = event-data() -> ("NewVal"=w136:u16)  [unwired: 1 out]
            n99 = property on="LaserJob" class="Ring (strict)"() -> ("Strings []"=w142:string[])  [unwired: 2 in, 2 out]
            n100 = Index Array(array=w142, index=w136) -> (element=w138:string)
            n101 = case shown="Default" w137 {
              tunnel: w140 -> [w149 w154]
              tunnel: [w148 w153] -> w139
              tunnel: w138 -> [w147 w152]
              tunnel: Station.Changeover.State.vi."NOK" ("State") -> [w146 w151]
              tunnel: w136 -> [w145 w150]
              frame Default {
                n102 = Bundle By Name(cluster=w149, "State"=w146, "Wabco.LaserJob"=w147, "Wabco.ScannerProgram"=w145) -> (w148:T3)
              }
              frame "Client" {
                n103 = Bundle By Name(cluster=w154, "State"=w151, "Client.LaserJob"=w152, "Client.ScannerProgram"=w150) -> (w153:T3)
              }
            }
            n104 = call "citTemplate.writeQueue.vi"("event in (if not connected:all statemachine with data event)"=ChangeOverGui.Action."Check" ("Action")) -> ()  [unwired: 14 in, 1 out]
          }
          event Value Change {
            n105 = event-data() -> ("NewVal"=w157:string)  [unwired: 1 out]
            n106 = case shown="\"Client\"" w155 {
              tunnel: w160 -> [w165 w169]
              tunnel: [w164 w168] -> w159
              tunnel: w157 -> [w163 w167]
              tunnel: Station.Changeover.State.vi."NOK" ("State") -> [w162 w166]
              frame Default {
                n107 = Bundle By Name(cluster=w165, "State"=w162, "Wabco.AdditionalTxt"=w163) -> (w164:T3)
              }
              frame "Client" {
                n108 = Bundle By Name(cluster=w169, "State"=w166, "Client.AdditionalTxt"=w167) -> (w168:T3)
              }
            }
            n109 = call "citTemplate.writeQueue.vi"("event in (if not connected:all statemachine with data event)"=ChangeOverGui.Action."Check" ("Action")) -> ()  [unwired: 14 in, 1 out]
          }
          event Value Change {
            n110 = event-data() -> ("NewVal"=w170:string)  [unwired: 1 out]
            n111 = case shown="Default" w172 {
              tunnel: w174 -> [w180 w184]
              tunnel: [w179 w183] -> w173
              tunnel: w170 -> [w178 w182]
              tunnel: Station.Changeover.State.vi."NOK" ("State") -> [w177 w181]
              frame Default {
                n112 = Bundle By Name(cluster=w180, "State"=w177, "Wabco.FactoryCode"=w178) -> (w179:T3)
              }
              frame "Client" {
                n113 = Bundle By Name(cluster=w184, "State"=w181, "Client.FactoryCode"=w182) -> (w183:T3)
              }
            }
            n114 = call "citTemplate.writeQueue.vi"("event in (if not connected:all statemachine with data event)"=ChangeOverGui.Action."Check" ("Action")) -> ()  [unwired: 14 in, 1 out]
          }
          event Value Change {
            n115 = event-data() -> ("NewVal"=w186:u8)  [unwired: 1 out]
            n116 = case shown="Default" w187 {
              tunnel: w189 -> [w195 w199]
              tunnel: [w194 w198] -> w188
              tunnel: w186 -> [w193 w197]
              tunnel: Station.Changeover.State.vi."NOK" ("State") -> [w192 w196]
              frame Default {
                n117 = Bundle By Name(cluster=w195, "State"=w192, "Wabco.RevID"=w193) -> (w194:T3)
              }
              frame "Client" {
                n118 = Bundle By Name(cluster=w199, "State"=w196, "Client.RevID"=w197) -> (w198:T3)
              }
            }
            n119 = call "citTemplate.writeQueue.vi"("event in (if not connected:all statemachine with data event)"=ChangeOverGui.Action."Check" ("Action")) -> ()  [unwired: 14 in, 1 out]
          }
          event Value Change {
            n120 = event-data() -> ("NewVal"=w200:u8)  [unwired: 1 out]
            n121 = case shown="\"Client\"" w202 {
              tunnel: w204 -> [w210 w214]
              tunnel: [w209 w213] -> w203
              tunnel: w200 -> [w208 w212]
              tunnel: Station.Changeover.State.vi."NOK" ("State") -> [w207 w211]
              frame Default {
                n122 = Bundle By Name(cluster=w210, "State"=w207, "Wabco.ForkID"=w208) -> (w209:T3)
              }
              frame "Client" {
                n123 = Bundle By Name(cluster=w214, "State"=w211, "Client.ForkID"=w212) -> (w213:T3)
              }
            }
            n124 = call "citTemplate.writeQueue.vi"("event in (if not connected:all statemachine with data event)"=ChangeOverGui.Action."Check" ("Action")) -> ()  [unwired: 14 in, 1 out]
          }
          event Value Change {
            n125 = event-data() -> ("NewVal"=w215:u16)  [unwired: 1 out]
            n126 = case shown="Default" w216 {
              tunnel: w218 -> [w225 w229]
              tunnel: [w224 w228] -> w217
              tunnel: w215 -> [w223 w227]
              tunnel: Station.Changeover.State.vi."NOK" ("State") -> [w222 w226]
              frame Default {
                n127 = Bundle By Name(cluster=w225, "State"=w222, "Wabco.FailuresLimit"=w223) -> (w224:T3)
              }
              frame "Client" {
                n128 = Bundle By Name(cluster=w229, "State"=w226, "Client.FailuresLimit"=w227) -> (w228:T3)
              }
            }
            n129 = call "citTemplate.writeQueue.vi"("event in (if not connected:all statemachine with data event)"=ChangeOverGui.Action."Check" ("Action")) -> ()  [unwired: 14 in, 1 out]
          }
          event Value Change {
            n130 = event-data() -> ("NewVal"=w231:i32)  [unwired: 1 out]
            n131 = case shown="\"Client\"" w230 {
              tunnel: w233 -> [w240 w244]
              tunnel: [w239 w243] -> w232
              tunnel: w231 -> [w238 w242]
              tunnel: Station.Changeover.State.vi."NOK" ("State") -> [w237 w241]
              frame Default {
                n132 = Bundle By Name(cluster=w240, "State"=w237, "Wabco.GlobalCnt"=w238) -> (w239:T3)
              }
              frame "Client" {
                n133 = Bundle By Name(cluster=w244, "State"=w241, "Client.GlobalCnt"=w242) -> (w243:T3)
              }
            }
            n134 = call "citTemplate.writeQueue.vi"("event in (if not connected:all statemachine with data event)"=ChangeOverGui.Action."Check" ("Action")) -> ()  [unwired: 14 in, 1 out]
          }
          event Value Change {
            n135 = event-data() -> ("NewVal"=w245:enum8{"A/B-1", "A/B-2", "A/B-3"})  [unwired: 1 out]
            n136 = case shown="\"Client\"" w247 {
              tunnel: w248 -> [w255 w259]
              tunnel: [w254 w258] -> w246
              tunnel: w245 -> [w253 w257]
              tunnel: Station.Changeover.State.vi."NOK" ("State") -> [w252 w256]
              frame Default {
                n137 = Bundle By Name(cluster=w255, "State"=w252, "Wabco.ScannerProgram"=w253) -> (w254:T3)
              }
              frame "Client" {
                n138 = Bundle By Name(cluster=w259, "State"=w256, "Client.ScannerProgram"=w257) -> (w258:T3)
              }
            }
            n139 = call "citTemplate.writeQueue.vi"("event in (if not connected:all statemachine with data event)"=ChangeOverGui.Action."Check" ("Action")) -> ()  [unwired: 14 in, 1 out]
          }
          event Value Change {
            n140 = event-data() -> ("NewVal"=w261:enum16{"", "6 dig", "7 dig"})  [unwired: 1 out]
            n141 = case shown="Default" w260 {
              tunnel: w263 -> [w270 w274]
              tunnel: [w269 w273] -> w262
              tunnel: w261 -> [w268 w272]
              tunnel: Station.Changeover.State.vi."NOK" ("State") -> [w267 w271]
              frame Default {
                n142 = Bundle By Name(cluster=w270, "State"=w267, "Wabco.SerialFormat"=w268) -> (w269:T3)
              }
              frame "Client" {
                n143 = Bundle By Name(cluster=w274, "State"=w271, "Client.SerialFormat"=w272) -> (w273:T3)
              }
            }
            n144 = call "citTemplate.writeQueue.vi"("event in (if not connected:all statemachine with data event)"=ChangeOverGui.Action."Check" ("Action")) -> ()  [unwired: 14 in, 1 out]
          }
          event Value Change {
            n145 = event-data() -> ("NewVal"=w276:cluster{"X":dbl, "Y":dbl, "Angle":dbl})  [unwired: 1 out]
            n146 = case shown="Default" w277 {
              tunnel: w278 -> [w285 w289]
              tunnel: [w284 w288] -> w275
              tunnel: w276 -> [w283 w287]
              tunnel: Station.Changeover.State.vi."NOK" ("State") -> [w282 w286]
              frame Default {
                n147 = Bundle By Name(cluster=w285, "State"=w282, "Wabco.CoordA"=w283) -> (w284:T3)
              }
              frame "Client" {
                n148 = Bundle By Name(cluster=w289, "State"=w286, "Client.CoordA"=w287) -> (w288:T3)
              }
            }
            n149 = call "citTemplate.writeQueue.vi"("event in (if not connected:all statemachine with data event)"=ChangeOverGui.Action."Check" ("Action")) -> ()  [unwired: 14 in, 1 out]
          }
          event Value Change {
            n150 = event-data() -> ("NewVal"=w291:cluster{"X":dbl, "Y":dbl, "Angle":dbl})  [unwired: 1 out]
            n151 = case shown="Default" w292 {
              tunnel: w293 -> [w300 w304]
              tunnel: [w299 w303] -> w290
              tunnel: w291 -> [w298 w302]
              tunnel: Station.Changeover.State.vi."NOK" ("State") -> [w297 w301]
              frame Default {
                n152 = Bundle By Name(cluster=w300, "State"=w297, "Wabco.CoordB"=w298) -> (w299:T3)
              }
              frame "Client" {
                n153 = Bundle By Name(cluster=w304, "State"=w301, "Client.CoordB"=w302) -> (w303:T3)
              }
            }
            n154 = call "citTemplate.writeQueue.vi"("event in (if not connected:all statemachine with data event)"=ChangeOverGui.Action."Check" ("Action")) -> ()  [unwired: 14 in, 1 out]
          }
          event Value Change {
            n155 = event-data() -> ()  [unwired: 2 out]
            n156 = case shown="\"Client\"" w305 {
              tunnel: [Sequence.PlateType."Client" ("Plate") Sequence.PlateType."Wabco" ("Plate")] -> w306
              frame "Client" {
              }
              frame Default {
              }
            }
            n157 = call "DMCConfiguratorGui-Open.vi"("error in"=w312, "Plate"=w306, "OrderSets"=w310) -> ("error out"=w311:errorcluster)  [unwired: 8 in]
            n158 = local read "Properties"() -> (w307:T1)
            n159 = Bundle By Name(cluster=w307, "SetupDMC"=FALSE) -> (w308:T1)
            n160 = call "MainGui-ModeSelect.vi"("error in (no error)"=w311, "Mode"=Sequence.MainMode."DMC Config") -> ("error out"=w314:errorcluster)  [unwired: 9 in]
            n161 = local write "Properties"(w308) -> ()
          }
          event Value Change {
            n162 = event-data() -> ("NewVal"=w319:u8)  [unwired: 1 out]
            n163 = case shown="\"Wabco\"" w320 {
              tunnel: w321 -> [w326 w330]
              tunnel: w319 -> [w325 w329]
              tunnel: Station.Changeover.State.vi."NOK" ("State") -> [w324 w328]
              tunnel: [w323 w327] -> w317
              frame "Wabco" {
                n164 = Bundle By Name(cluster=w326, "State"=w324, "Wabco.CVX_Program"=w325) -> (w323:T3)
              }
              frame "Client", Default {
                n165 = Bundle By Name(cluster=w330, "State"=w328, "Client.CVX_Program"=w329) -> (w327:T3)
              }
            }
          }
        }
      }
      frame "constructor" {
        n166 = stacked-sequence {
          tunnel: w334 -> [w338 _ _]
          tunnel: [w345 _ _] -> w333
          tunnel: w332 -> [_ _ _]
          tunnel: [_ w366 _] -> w331
          frame #0 {
            w336 = TRUE ("Visible")
            w339 = T28 {"Width"=200, "Height"=200} ("Draw Area Size")
            n167 = property on="StartHere..." class="Bool (strict)"() -> (error out=w347:errorcluster, "Position"=w346:T29)  [unwired: 2 in, 1 out]
            n168 = control-ref of="This VI"() -> (w348:refnum<vi>)
            n169 = property class="VI"(reference=w348) -> (reference out=w344:refnum<vi>, error out=w342:errorcluster, "Front Panel"=→"Panel":refnum<vi>, "FP.State"=w341:T18)  [unwired: 1 in]
            n170 = property on="Pane" class="Pane"(error in=w347, "Origin"=w346) -> ()  [unwired: 1 in, 2 out]
            n171 = property on="Properties" class="Clust (strict)"(error in=w338, "Visible"=w336) -> (error out=w337:errorcluster)  [unwired: 1 in, 1 out]
            n172 = case shown="\"Standard\", \"Minimized\", \"Maximized\"" w341 {
              tunnel: w344 -> [w351 w355]
              tunnel: w342 -> [w350 w354]
              tunnel: [w351 w353] -> w343
              tunnel: [w350 w352] -> _
              frame Default {
              }
              frame "Standard", "Minimized", "Maximized" {
                n173 = invoke class="VI" method="FP.Close"(reference=w355, error in=w354) -> (reference out=w353:refnum<vi>, error out=w352:errorcluster)  [unwired: 1 in, 1 out]
              }
            }
            n174 = property on="OrdersTable" class="MCListbox (strict)"(error in=w337, "Visible"=w336) -> (error out=w335:errorcluster)  [unwired: 1 in, 1 out]
            n175 = property on="WabcoPlate" class="Pict"("Draw Area Size"=w339) -> (error out=w340:errorcluster)  [unwired: 2 in, 1 out]
            n176 = global write "ApplicationGlobal.vi" "GuiRef.ChangeOver"(w343) -> ()
            n177 = property on="ClientPlate" class="Pict"(error in=w340, "Draw Area Size"=w339) -> ()  [unwired: 1 in, 2 out]
            n178 = call "Translator.TranslateThis.Init.vi"("error in"=w335) -> ("error out"=w345:errorcluster)  [unwired: 10 in]
          }
          frame #1 {
            w356 = FALSE ("Visible")
            w363 = picture data[5B] ("picture")
            n179 = global read "Sequence.Global.vi" "SeqData"() -> (w362:T30)
            n180 = property on="Properties" class="Clust (strict)"("Visible"=w356) -> ()  [unwired: 2 in, 2 out]
            n181 = Unbundle By Name(w362) -> ("Code.Variant"=w364:T3, "Status.Process"=w365:T31)
            n182 = property on="OrdersTable" class="MCListbox (strict)"("Visible"=w356) -> ()  [unwired: 2 in, 2 out]
            n183 = call "citTemplate.writeQueue.vi"("event in (if not connected:all statemachine with data event)"=ChangeOverGui.Action."Clear" ("Action")) -> ("error out"=w360:errorcluster)  [unwired: 14 in]
            n184 = case shown="\"Pending\", \"Running\", \"Error\"..\"Stopped\"" w365 {
              tunnel: [w368 w369] -> w366
              tunnel: w364 -> [w368 w369]
              tunnel: w360 -> [_ _]
              frame "Pending", "Running", "Error".."Stopped" {
                n185 = call "citTemplate.writeQueue.vi"("event in (if not connected:all statemachine with data event)"=ChangeOverGui.Action."Read File" ("Action")) -> ()  [unwired: 14 in, 1 out]
              }
              frame Default {
                n186 = call "ChangeOverGui-RefReject.vi"() -> ()  [unwired: 11 in, 1 out]
              }
            }
            n187 = local write "Image"(w363) -> ()
            n188 = local write "WabcoPlate"(w363) -> ()
            n189 = local write "ClientPlate"(w363) -> ()
            n190 = property on="OrdersTable" class="MCListbox (strict)"("ItemNames"=string[][] [] ("Item Names"), "Value"=0 ("OrdersTable"), "TopLeft"=T12 {"Row"=0, "Column"=0} ("Top Left Visible Cell")) -> ()  [unwired: 2 in, 2 out]
          }
          frame #2 {
            n191 = while {
              stop <- w371 stop-if-true
              n192 = global read "ApplicationGlobal.vi" "AppLaunched"() -> (w371:bool)
              n193 = Wait (ms)(milliseconds to wait=u32 50) -> ()  [unwired: 1 out]
            }
          }
        }
      }
      frame "destructor" {
        n194 = local read "Panel"() -> (w373:refnum<vi>)
        n195 = property class="Pnl"(reference=w373, "DeferPanUpdts"=FALSE ("Defer Panel Updates")) -> (reference out=w375:refnum<vi>, error out=w376:errorcluster)  [unwired: 1 in]
        n196 = call "Translator.TranslateThis.Exit.vi"("error in"=w378) -> ("error out"=w377:errorcluster)  [unwired: 10 in]
        n197 = Close Reference(reference=w375, error in (no error)=w376) -> ()  [unwired: 1 out]
      }
      frame "---ChangeOverGui ---" {
        w384 = EventLog.EventSource."Ref" ("Event source")
        n198 = Unflatten From String(type=T13 {"ts"=timestamp(0 s since 1904-01-01), "src"=enum."All", "instance"=0, "action"="", "error"={"status"=FALSE, "code"=0, "source"=""}, "unconfirmed"=FALSE} ("ErrData"), binary string=w388, error in (no error)=w387) -> (value=w382:T13, error out=w383:errorcluster)  [unwired: 3 out]
        n199 = call "ErrorHandling.Fglb.Add.vi"("Event source"=w384, "error in (no error)"=w383, "Error in"=w382) -> ("error out"=w386:errorcluster, "changed?"=w385:bool)  [unwired: 7 in]
        n200 = case shown="True" w385 {
          tunnel: [w390 w394] -> w381
          tunnel: w382 -> [_ w393]
          tunnel: w386 -> [w390 w392]
          tunnel: w384 -> [_ w391]
          frame False {
          }
          frame True {
            n201 = call "EventLog.New(error).vi"("Source (All)"=w391, "error in"=w392, "ErrData"=w393) -> ("error out"=w394:errorcluster)  [unwired: 8 in]
          }
        }
      }
      frame "Clear" {
        w397 = FALSE ("Visible")
        w401 = FALSE ("Blinking")
        w395 = FALSE ("Blinking")
        n202 = property on="ProductNo" class="Str"("Blinking"=w395) -> (error out=w418:errorcluster)  [unwired: 2 in, 1 out]
        n203 = property on="ShowPropertiesWabco" class="Bool (strict)"("Value"=w401, "Blinking"=w401) -> (error out=w404:errorcluster)  [unwired: 2 in, 1 out]
        n204 = property on="PlateNo" class="Str"(error in=w418, "Blinking"=w395) -> (error out=w417:errorcluster)  [unwired: 1 in, 1 out]
        n205 = property on="ProductNo" class="Str"(error in=w417, "Blinking"=w395) -> (error out=w416:errorcluster)  [unwired: 1 in, 1 out]
        n206 = property on="ShowPropertiesClient" class="Bool (strict)"(error in=w404, "Value"=w401, "Blinking"=w401) -> (error out=w403:errorcluster)  [unwired: 1 in, 1 out]
        n207 = property on="PlateNo" class="Str"(error in=w416, "Blinking"=w395) -> (error out=w415:errorcluster)  [unwired: 1 in, 1 out]
        n208 = property on="TotalQuantity" class="DigNum (strict)"(error in=w415, "Blinking"=w395) -> (error out=w414:errorcluster)  [unwired: 1 in, 1 out]
        n209 = property on="ViewMode" class="Enum (strict)"(error in=w403, "Value"=0) -> (error out=w402:errorcluster)  [unwired: 1 in, 1 out]
        n210 = property on="SerialNo" class="DigNum (strict)"(error in=w414, "Blinking"=w395) -> (error out=w413:errorcluster)  [unwired: 1 in, 1 out]
        n211 = property on="LaserJob" class="Ring (strict)"(error in=w413, "Blinking"=w395) -> (error out=w411:errorcluster)  [unwired: 1 in, 1 out]
        n212 = property on="Properties" class="Clust (strict)"(error in=w402, "Visible"=w397) -> (error out=w398:errorcluster)  [unwired: 1 in, 1 out]
        n213 = call "citTemplate.writeQueue.vi"("event in (if not connected:all statemachine with data event)"=ChangeOverGui.Action."Check" ("Action")) -> ()  [unwired: 14 in, 1 out]
        n214 = property on="RevID" class="DigNum (strict)"(error in=w411, "Blinking"=w395) -> (error out=w412:errorcluster)  [unwired: 1 in, 1 out]
        n215 = property on="ShowOrdersTable" class="Bool (strict)"(error in=w398, "Value"=w397) -> (error out=w399:errorcluster)  [unwired: 1 in, 1 out]
        n216 = property on="ForkID" class="DigNum (strict)"(error in=w412, "Blinking"=w395) -> (error out=w419:errorcluster)  [unwired: 1 in, 1 out]
        n217 = property on="FactoryCode" class="Str"("Blinking"=w395) -> ()  [unwired: 2 in, 2 out]
        n218 = property on="X" class="DigNum (strict)"(error in=w419, "Blinking"=w395) -> (error out=w410:errorcluster)  [unwired: 1 in, 1 out]
        n219 = property on="OrdersTable" class="MCListbox (strict)"(error in=w399, "Visible"=w397) -> (error out=w396:errorcluster)  [unwired: 1 in, 1 out]
        n220 = property on="Y" class="DigNum (strict)"(error in=w410, "Blinking"=w395) -> (error out=w409:errorcluster)  [unwired: 1 in, 1 out]
        n221 = property on="SetupDMC" class="Bool (strict)"("Blinking"=w395) -> ()  [unwired: 2 in, 2 out]
        n222 = property on="Progress" class="Bool (strict)"(error in=w396, "Visible"=w397) -> ()  [unwired: 1 in, 2 out]
        n223 = property on="Angle" class="DigNum (strict)"(error in=w409, "Blinking"=w395) -> (error out=w406:errorcluster)  [unwired: 1 in, 1 out]
        n224 = property on="X" class="DigNum (strict)"(error in=w406, "Blinking"=w395) -> (error out=w407:errorcluster)  [unwired: 1 in, 1 out]
        n225 = property on="Y" class="DigNum (strict)"(error in=w407, "Blinking"=w395) -> (error out=w408:errorcluster)  [unwired: 1 in, 1 out]
        n226 = property on="Angle" class="DigNum (strict)"(error in=w408, "Blinking"=w395) -> ()  [unwired: 1 in, 2 out]
      }
      frame "Validate" {
        n227 = local read "DoubleOrder"() -> (w422:bool)
        n228 = Unbundle By Name(w426) -> ("State"=w427:T4)
        n229 = case shown="\"NOK\", \"Wait for ack\"" w427 {
          selector: w427 -> [w429 w445]
          tunnel: w426 -> [_ w442]
          tunnel: [w429 w441] -> w424
          tunnel: w423 -> [_ w438]
          tunnel: w422 -> [_ w437]
          frame Default {
          }
          frame "NOK", "Wait for ack" {
            n230 = while {
              tunnel: [w454] -> w434 mode=indexing
              tunnel: w442 -> [w452]
              tunnel: w438 -> [w451]
              tunnel: w437 -> [w450]
              i -> [w455]
              stop <- w453 stop-if-true
              n231 = case shown="10" w455 {
                tunnel: [w456 w460 _ _ w469 w472 w473 w489 w497 w502 w505 w516 w523 w532 w542 w549 w556 w575 w591 w598 w605 w615 w628 w637 w647 w659 w666 _] -> w454
                tunnel: w452 -> [w459 w463 w465 w466 w468 w471 w475 w492 w495 w500 w511 w515 w528 w537 w541 w554 w568 w574 w593 w600 w613 w620 w633 w644 w651 w664 w678 _]
                tunnel: [_ _ _ _ _ _ _ _ _ _ _ _ _ _ _ _ _ _ _ _ _ _ _ _ _ _ _ TRUE] -> w453
                tunnel: w451 -> [_ _ _ _ _ _ w474 w491 w494 w499 w504 w514 w522 w530 w540 w548 w565 w573 w592 w599 w607 w619 w629 w638 w650 w660 w667 _]
                tunnel: w450 -> [_ _ _ _ _ _ _ _ _ _ _ _ _ _ _ _ _ w572 w590 w597 w606 w616 w626 w635 w646 w657 _ _]
                frame 0 {
                  n232 = Unbundle By Name(w459) -> ("WabcoPlate"=w458:string)
                  n233 = call "ChangeOverGui.RefNumFormatStr.vi"("RefNum in"=w458) -> ("RefNum format ok?"=w457:bool)  [unwired: 2 out]
                  n234 = Not(x=w457) -> (.not. x?=w456:bool)
                  n235 = property on="PlateNo" class="Str"("Blinking"=w456) -> ()  [unwired: 2 in, 2 out]
                }
                frame 1 {
                  n236 = Unbundle By Name(w463) -> ("WabcoProduct"=w462:string)
                  n237 = call "ChangeOverGui.RefNumFormatStr.vi"("RefNum in"=w462) -> ("RefNum format ok?"=w461:bool)  [unwired: 2 out]
                  n238 = Not(x=w461) -> (.not. x?=w460:bool)
                  n239 = property on="ProductNo" class="Str"("Blinking"=w460) -> ()  [unwired: 2 in, 2 out]
                }
                frame 2 {
                  n240 = Unbundle By Name(w465) -> ("ClientPlate"=w464:string)
                  n241 = call "ChangeOverGui.RefNumFormatStr.vi"("RefNum in"=w464) -> ()  [unwired: 3 out]
                }
                frame 3 {
                  n242 = Unbundle By Name(w466) -> ()  [unwired: 1 out]
                }
                frame 4 {
                  n243 = Unbundle By Name(w468) -> ("TotalQuantity"=w467:u16)
                  n244 = Less Or Equal To 0?(x=w467) -> (x <= 0?=w469:bool)
                  n245 = property on="TotalQuantity" class="DigNum (strict)"("Blinking"=w469) -> ()  [unwired: 2 in, 2 out]
                }
                frame 5 {
                  n246 = Unbundle By Name(w471) -> ("Serial"=w470:i32)
                  n247 = Less Than 0?(x=w470) -> (x < 0?=w472:bool)
                  n248 = property on="SerialNo" class="DigNum (strict)"("Blinking"=w472) -> ()  [unwired: 2 in, 2 out]
                }
                frame 6 {
                  n249 = global read "V7310.Global.vi" "Laser.Status"() -> (w479:T39)
                  n250 = Unbundle By Name(w475) -> ("Wabco.LaserJob"=w487:string)
                  n251 = property on="LaserJob" class="Ring (strict)"() -> ("Strings []"=w477:string[], "Value"=w481:u16)  [unwired: 2 in, 2 out]
                  n252 = Unbundle By Name(w479) -> ("Jobs"=w480:string[])
                  n253 = Index Array(array=w477, index=w481) -> (element=w482:string)
                  n254 = Build Array (concatenate)("", w480) -> (w476:string[])
                  n255 = Search 1D Array(1D array=w476, element=w487) -> (index of element=w486:i32)  [unwired: 1 in]
                  n256 = Search 1D Array(1D array=w476, element=w482) -> (index of element=w483:i32)  [unwired: 1 in]
                  n257 = Less Or Equal To 0?(x=w486) -> (x <= 0?=w473:bool)
                  n258 = Max & Min(x=w483, y=0) -> (max(x,y)=w485:i32)  [unwired: 1 out]
                  n259 = case shown="\"Wabco\"" w474 {
                    tunnel: w473 -> [w488 _]
                    frame "Wabco" {
                      n260 = property on="LaserJob" class="Ring (strict)"("Blinking"=w488) -> ()  [unwired: 2 in, 2 out]
                    }
                    frame Default {
                    }
                  }
                  n261 = property on="LaserJob" class="Ring (strict)"("Strings []"=w476, "Value"=w485) -> ()  [unwired: 2 in, 2 out]
                }
                frame 7 {
                  n262 = Unbundle By Name(w492) -> ("Wabco.FactoryCode"=w490:string)
                  n263 = Empty String/Path?(string/path=w490) -> (empty?=w489:bool)
                  n264 = case shown="\"Wabco\"" w491 {
                    tunnel: w489 -> [w493 _]
                    frame "Wabco" {
                      n265 = property on="FactoryCode" class="Str"("Blinking"=w493) -> ()  [unwired: 2 in, 2 out]
                    }
                    frame Default {
                    }
                  }
                }
                frame 8 {
                  n266 = Unbundle By Name(w495) -> ("Wabco.RevID"=w496:u8)
                  n267 = Less Or Equal To 0?(x=w496) -> (x <= 0?=w497:bool)
                  n268 = case shown="\"Wabco\"" w494 {
                    tunnel: w497 -> [_ w498]
                    frame Default {
                    }
                    frame "Wabco" {
                      n269 = property on="RevID" class="DigNum (strict)"("Blinking"=w498) -> ()  [unwired: 2 in, 2 out]
                    }
                  }
                }
                frame 9 {
                  n270 = Unbundle By Name(w500) -> ("Wabco.ForkID"=w501:u8)
                  n271 = Less Or Equal To 0?(x=w501) -> (x <= 0?=w502:bool)
                  n272 = case shown="\"Wabco\"" w499 {
                    tunnel: w502 -> [_ w503]
                    frame Default {
                    }
                    frame "Wabco" {
                      n273 = property on="ForkID" class="DigNum (strict)"("Blinking"=w503) -> ()  [unwired: 2 in, 2 out]
                    }
                  }
                }
                frame 10 {
                  n274 = Unbundle By Name(w511) -> ("Wabco.CoordA.X"=w507:dbl)
                  n275 = Not Equal To 0?(x=w507) -> (x != 0?=w506:bool)
                  n276 = In Range and Coerce(upper limit=45.0 ("CoordinateA-Angle"), x=w507, lower limit=-45.0 ("CoordinateA-Angle")) -> (In Range?=w508:bool)  [unwired: 1 out]
                  n277 = Compound Arithmetic op=AND(w508, w506) -> (invert w505:bool)
                  n278 = case shown="\"Wabco\"" w504 {
                    tunnel: w505 -> [_ w512]
                    frame Default {
                    }
                    frame "Wabco" {
                      n279 = property on="X" class="DigNum (strict)"("Blinking"=w512) -> ()  [unwired: 2 in, 2 out]
                    }
                  }
                }
                frame 11 {
                  n280 = Unbundle By Name(w515) -> ("Wabco.CoordA.Y"=w513:dbl)
                  n281 = Not Equal To 0?(x=w513) -> (x != 0?=w517:bool)
                  n282 = In Range and Coerce(upper limit=45.0 ("CoordinateA-Angle"), x=w513, lower limit=-45.0 ("CoordinateA-Angle")) -> (In Range?=w518:bool)  [unwired: 1 out]
                  n283 = Compound Arithmetic op=AND(w518, w517) -> (invert w516:bool)
                  n284 = case shown="\"Wabco\"" w514 {
                    tunnel: w516 -> [_ w521]
                    frame Default {
                    }
                    frame "Wabco" {
                      n285 = property on="Y" class="DigNum (strict)"("Blinking"=w521) -> ()  [unwired: 2 in, 2 out]
                    }
                  }
                }
                frame 12 {
                  n286 = Unbundle By Name(w528) -> ("Wabco.CoordA.Angle"=w527:dbl)
                  n287 = In Range and Coerce(upper limit=180.0 ("CoordinateA-Angle"), x=w527, lower limit=-180.0 ("CoordinateA-Angle")) -> (In Range?=w524:bool)  [unwired: 1 out]
                  n288 = Not(x=w524) -> (.not. x?=w523:bool)
                  n289 = case shown="\"Wabco\"" w522 {
                    tunnel: w523 -> [_ w529]
                    frame Default {
                    }
                    frame "Wabco" {
                      n290 = property on="Angle" class="DigNum (strict)"("Blinking"=w529) -> ()  [unwired: 2 in, 2 out]
                    }
                  }
                }
                frame 13 {
                  n291 = Unbundle By Name(w537) -> ("Wabco.CoordB.X"=w531:dbl)
                  n292 = Not Equal To 0?(x=w531) -> (x != 0?=w533:bool)
                  n293 = In Range and Coerce(upper limit=45.0 ("CoordinateA-Angle"), x=w531, lower limit=-45.0 ("CoordinateA-Angle")) -> (In Range?=w534:bool)  [unwired: 1 out]
                  n294 = Compound Arithmetic op=AND(w534, w533) -> (invert w532:bool)
                  n295 = case shown="\"Wabco\"" w530 {
                    tunnel: w532 -> [_ w538]
                    frame Default {
                    }
                    frame "Wabco" {
                      n296 = property on="X" class="DigNum (strict)"("Blinking"=w538) -> ()  [unwired: 2 in, 2 out]
                    }
                  }
                }
                frame 14 {
                  n297 = Unbundle By Name(w541) -> ("Wabco.CoordB.Y"=w539:dbl)
                  n298 = Not Equal To 0?(x=w539) -> (x != 0?=w543:bool)
                  n299 = In Range and Coerce(upper limit=45.0 ("CoordinateA-Angle"), x=w539, lower limit=-45.0 ("CoordinateA-Angle")) -> (In Range?=w544:bool)  [unwired: 1 out]
                  n300 = Compound Arithmetic op=AND(w544, w543) -> (invert w542:bool)
                  n301 = case shown="\"Wabco\"" w540 {
                    tunnel: w542 -> [_ w547]
                    frame Default {
                    }
                    frame "Wabco" {
                      n302 = property on="Y" class="DigNum (strict)"("Blinking"=w547) -> ()  [unwired: 2 in, 2 out]
                    }
                  }
                }
                frame 15 {
                  n303 = Unbundle By Name(w554) -> ("Wabco.CoordB.Angle"=w553:dbl)
                  n304 = In Range and Coerce(upper limit=180.0 ("CoordinateA-Angle"), x=w553, lower limit=-180.0 ("CoordinateA-Angle")) -> (In Range?=w550:bool)  [unwired: 1 out]
                  n305 = Not(x=w550) -> (.not. x?=w549:bool)
                  n306 = case shown="\"Wabco\"" w548 {
                    tunnel: w549 -> [_ w555]
                    frame Default {
                    }
                    frame "Wabco" {
                      n307 = property on="Angle" class="DigNum (strict)"("Blinking"=w555) -> ()  [unwired: 2 in, 2 out]
                    }
                  }
                }
                frame 16 {
                  n308 = Unbundle By Name(w568) -> ("Wabco.DMCconfig"=w564:i32, "Wabco.GlobalCnt"=w567:i32)
                  n309 = global read "Station.Global.vi" "DMCdata"() -> (w557:T44[])
                  n310 = Equal To 0?(x=w564) -> (x = 0?=w566:bool)
                  n311 = Index Array(array=w557, index=w564) -> (element=w563:T44)
                  n312 = Greater Than 0?(x=w564) -> (x > 0?=w562:bool)
                  n313 = call "Sequence.Test.CreateDMC.vi"("Default"=w566, "Serial (0)"=w567, "DMCConfig"=w563, "Plate"=Sequence.PlateType."Wabco", "Variant"=w568) -> ("DMC nok"=w558:bool)  [unwired: 5 in, 1 out]
                  n314 = Select(t=u32 16711680, s=w562, f=u32 0) -> (s? t:f=w559:u32)
                  n315 = case shown="Default" w565 {
                    tunnel: w558 -> [_ w570]
                    tunnel: w559 -> [_ w571]
                    tunnel: [_ w570] -> w556
                    frame Default {
                    }
                    frame "Wabco" {
                      n316 = property on="SetupDMC" class="Bool (strict)"("Blinking"=w570, "BoolText.TextColor"=w571) -> ()  [unwired: 2 in, 2 out]
                    }
                  }
                }
                frame 17 {
                  n317 = global read "V7310.Global.vi" "Laser.Status"() -> (w579:T39)
                  n318 = Unbundle By Name(w574) -> ("Client.LaserJob"=w588:string)
                  n319 = property on="LaserJob" class="Ring (strict)"() -> ("Strings []"=w577:string[], "Value"=w581:u16)  [unwired: 2 in, 2 out]
                  n320 = Unbundle By Name(w579) -> ("Jobs"=w580:string[])
                  n321 = Index Array(array=w577, index=w581) -> (element=w582:string)
                  n322 = Build Array (concatenate)("", w580) -> (w576:string[])
                  n323 = Search 1D Array(1D array=w576, element=w588) -> (index of element=w587:i32)  [unwired: 1 in]
                  n324 = Search 1D Array(1D array=w576, element=w582) -> (index of element=w583:i32)  [unwired: 1 in]
                  n325 = Less Or Equal To 0?(x=w587) -> (x <= 0?=w586:bool)
                  n326 = Compound Arithmetic op=AND(w586, w572) -> (w575:bool)
                  n327 = Max & Min(x=w583, y=0) -> (max(x,y)=w585:i32)  [unwired: 1 out]
                  n328 = case shown="\"Client\"" w573 {
                    tunnel: w575 -> [w589 _]
                    frame "Client" {
                      n329 = property on="LaserJob" class="Ring (strict)"("Blinking"=w589) -> ()  [unwired: 2 in, 2 out]
                    }
                    frame Default {
                    }
                  }
                  n330 = property on="LaserJob" class="Ring (strict)"("Strings []"=w576, "Value"=w585) -> ()  [unwired: 2 in, 2 out]
                }
                frame 18 {
                  n331 = Unbundle By Name(w593) -> ("Client.RevID"=w594:u8)
                  n332 = Less Or Equal To 0?(x=w594) -> (x <= 0?=w595:bool)
                  n333 = Compound Arithmetic op=AND(w595, w590) -> (w591:bool)
                  n334 = case shown="\"Client\"" w592 {
                    tunnel: w591 -> [_ w596]
                    frame Default {
                    }
                    frame "Client" {
                      n335 = property on="RevID" class="DigNum (strict)"("Blinking"=w596) -> ()  [unwired: 2 in, 2 out]
                    }
                  }
                }
                frame 19 {
                  n336 = Unbundle By Name(w600) -> ("Client.ForkID"=w601:u8)
                  n337 = Less Or Equal To 0?(x=w601) -> (x <= 0?=w602:bool)
                  n338 = Compound Arithmetic op=AND(w602, w597) -> (w598:bool)
                  n339 = case shown="\"Client\"" w599 {
                    tunnel: w598 -> [_ w603]
                    frame Default {
                    }
                    frame "Client" {
                      n340 = property on="ForkID" class="DigNum (strict)"("Blinking"=w603) -> ()  [unwired: 2 in, 2 out]
                    }
                  }
                }
                frame 20 {
                  n341 = Unbundle By Name(w613) -> ("Client.CoordA.X"=w609:dbl)
                  n342 = Not Equal To 0?(x=w609) -> (x != 0?=w608:bool)
                  n343 = In Range and Coerce(upper limit=45.0 ("CoordinateA-Angle"), x=w609, lower limit=-45.0 ("CoordinateA-Angle")) -> (In Range?=w610:bool)  [unwired: 1 out]
                  n344 = Compound Arithmetic op=AND(w610, w608) -> (invert w604:bool)
                  n345 = Compound Arithmetic op=AND(w604, w606) -> (w605:bool)
                  n346 = case shown="\"Client\"" w607 {
                    tunnel: w605 -> [_ w614]
                    frame Default {
                    }
                    frame "Client" {
                      n347 = property on="X" class="DigNum (strict)"("Blinking"=w614) -> ()  [unwired: 2 in, 2 out]
                    }
                  }
                }
                frame 21 {
                  n348 = Unbundle By Name(w620) -> ("Client.CoordA.Y"=w618:dbl)
                  n349 = Not Equal To 0?(x=w618) -> (x != 0?=w621:bool)
                  n350 = In Range and Coerce(upper limit=45.0 ("CoordinateA-Angle"), x=w618, lower limit=-45.0 ("CoordinateA-Angle")) -> (In Range?=w622:bool)  [unwired: 1 out]
                  n351 = Compound Arithmetic op=AND(w622, w621) -> (invert w617:bool)
                  n352 = Compound Arithmetic op=AND(w617, w616) -> (w615:bool)
                  n353 = case shown="\"Client\"" w619 {
                    tunnel: w615 -> [_ w625]
                    frame Default {
                    }
                    frame "Client" {
                      n354 = property on="Y" class="DigNum (strict)"("Blinking"=w625) -> ()  [unwired: 2 in, 2 out]
                    }
                  }
                }
                frame 22 {
                  n355 = Unbundle By Name(w633) -> ("Client.CoordA.Angle"=w632:dbl)
                  n356 = In Range and Coerce(upper limit=180.0 ("CoordinateA-Angle"), x=w632, lower limit=-180.0 ("CoordinateA-Angle")) -> (In Range?=w627:bool)  [unwired: 1 out]
                  n357 = Compound Arithmetic op=AND(invert w627, w626) -> (w628:bool)
                  n358 = case shown="\"Client\"" w629 {
                    tunnel: w628 -> [_ w634]
                    frame Default {
                    }
                    frame "Client" {
                      n359 = property on="Angle" class="DigNum (strict)"("Blinking"=w634) -> ()  [unwired: 2 in, 2 out]
                    }
                  }
                }
                frame 23 {
                  n360 = Unbundle By Name(w644) -> ("Client.CoordB.X"=w639:dbl)
                  n361 = Not Equal To 0?(x=w639) -> (x != 0?=w640:bool)
                  n362 = In Range and Coerce(upper limit=45.0 ("CoordinateA-Angle"), x=w639, lower limit=-45.0 ("CoordinateA-Angle")) -> (In Range?=w641:bool)  [unwired: 1 out]
                  n363 = Compound Arithmetic op=AND(w641, w640) -> (invert w636:bool)
                  n364 = Compound Arithmetic op=AND(w636, w635) -> (w637:bool)
                  n365 = case shown="\"Client\"" w638 {
                    tunnel: w637 -> [_ w645]
                    frame Default {
                    }
                    frame "Client" {
                      n366 = property on="X" class="DigNum (strict)"("Blinking"=w645) -> ()  [unwired: 2 in, 2 out]
                    }
                  }
                }
                frame 24 {
                  n367 = Unbundle By Name(w651) -> ("Client.CoordB.Y"=w649:dbl)
                  n368 = Not Equal To 0?(x=w649) -> (x != 0?=w652:bool)
                  n369 = In Range and Coerce(upper limit=45.0 ("CoordinateA-Angle"), x=w649, lower limit=-45.0 ("CoordinateA-Angle")) -> (In Range?=w653:bool)  [unwired: 1 out]
                  n370 = Compound Arithmetic op=AND(w653, w652) -> (invert w648:bool)
                  n371 = Compound Arithmetic op=AND(w648, w646) -> (w647:bool)
                  n372 = case shown="\"Client\"" w650 {
                    tunnel: w647 -> [_ w656]
                    frame Default {
                    }
                    frame "Client" {
                      n373 = property on="Y" class="DigNum (strict)"("Blinking"=w656) -> ()  [unwired: 2 in, 2 out]
                    }
                  }
                }
                frame 25 {
                  n374 = Unbundle By Name(w664) -> ("Client.CoordB.Angle"=w663:dbl)
                  n375 = In Range and Coerce(upper limit=180.0 ("CoordinateA-Angle"), x=w663, lower limit=-180.0 ("CoordinateA-Angle")) -> (In Range?=w658:bool)  [unwired: 1 out]
                  n376 = Compound Arithmetic op=AND(invert w658, w657) -> (w659:bool)
                  n377 = case shown="\"Client\"" w660 {
                    tunnel: w659 -> [_ w665]
                    frame Default {
                    }
                    frame "Client" {
                      n378 = property on="Angle" class="DigNum (strict)"("Blinking"=w665) -> ()  [unwired: 2 in, 2 out]
                    }
                  }
                }
                frame 26 {
                  n379 = Unbundle By Name(w678) -> ("Client.DMCconfig"=w675:i32, "Client.GlobalCnt"=w677:i32)
                  n380 = global read "Station.Global.vi" "DMCdata"() -> (w668:T44[])
                  n381 = Equal To 0?(x=w675) -> (x = 0?=w676:bool)
                  n382 = Index Array(array=w668, index=w675) -> (element=w674:T44)
                  n383 = Greater Than 0?(x=w675) -> (x > 0?=w673:bool)
                  n384 = call "Sequence.Test.CreateDMC.vi"("Default"=w676, "Serial (0)"=w677, "DMCConfig"=w674, "Plate"=Sequence.PlateType."Client", "Variant"=w678) -> ("DMC nok"=w669:bool)  [unwired: 5 in, 1 out]
                  n385 = Select(t=u32 16711680, s=w673, f=u32 0) -> (s? t:f=w670:u32)
                  n386 = case shown="\"Client\"" w667 {
                    tunnel: w669 -> [_ w680]
                    tunnel: w670 -> [_ w681]
                    tunnel: [_ w680] -> w666
                    frame Default {
                    }
                    frame "Client" {
                      n387 = property on="SetupDMC" class="Bool (strict)"("Blinking"=w680, "BoolText.TextColor"=w681) -> ()  [unwired: 2 in, 2 out]
                    }
                  }
                }
                frame Default {
                }
              }
            }
            n388 = Or Array Elements(Boolean array=w434) -> (logical OR=w448:bool)
            n389 = Array Subset(array=w434, index=6, length=11) -> (w435:bool[])
            n390 = Array Subset(array=w434, index=17, length=10) -> (w430:bool[])
            n391 = Select(t=Station.Changeover.State.vi."NOK" ("Changeover state"), s=w448, f=Station.Changeover.State.vi."Wait for ack" ("Changeover state")) -> (s? t:f=w441:T4)
            n392 = Or Array Elements(Boolean array=w435) -> (logical OR=w439:bool)
            n393 = Or Array Elements(Boolean array=w430) -> (logical OR=w431:bool)
            n394 = Not Equal?(x=w445, y=w441) -> (x != y?=w444:bool)
            n395 = property on="ShowPropertiesWabco" class="Bool (strict)"("Blinking"=w439) -> ()  [unwired: 2 in, 2 out]
            n396 = property on="ShowPropertiesClient" class="Bool (strict)"("Blinking"=w431) -> ()  [unwired: 2 in, 2 out]
            n397 = case shown="True" w444 {
              tunnel: ChangeOverGui.Action."Check" ("Action") -> [_ w449]
              frame False {
              }
              frame True {
                n398 = call "citTemplate.writeQueue.vi"("event in (if not connected:all statemachine with data event)"=w449) -> ()  [unwired: 14 in, 1 out]
              }
            }
          }
        }
        n399 = Bundle By Name(cluster=w426, "State"=w424) -> (w425:T3)
      }
      frame "Read File" {
        n400 = call "Logger.Variant.Read.vi"("error in (no error)"=w691, "VariantSets in"=w690) -> ("error out"=w688:errorcluster, "VariantSets out"=w689:T3, "OrdersTableIdx"=w685:i32, "OrdersTable"=w686:string[][])  [unwired: 4 in, 2 out]
        n401 = property on="OrdersTable" class="MCListbox (strict)"("ItemNames"=w686, "Value"=w685) -> ()  [unwired: 2 in, 2 out]
        n402 = call "citTemplate.writeQueue.vi"("event in (if not connected:all statemachine with data event)"=ChangeOverGui.Action."Update Table" ("Action")) -> ("error out"=w683:errorcluster)  [unwired: 14 in]
        n403 = call "citTemplate.writeQueue.vi"("event in (if not connected:all statemachine with data event)"=ChangeOverGui.Action."Read Imgs" ("Action"), "error in (no error)"=w683) -> ()  [unwired: 13 in, 1 out]
      }
      frame "Read Imgs" {
        n404 = global read "ApplicationGlobal.vi" "PlatesPath"() -> (w695:path)
        n405 = Unbundle By Name(w693) -> ("ImgPath"=w692:path)
        n406 = stacked-sequence {
          tunnel: w693 -> [_ w720 w739]
          tunnel: w695 -> [_ w726 w738]
          tunnel: w692 -> [w697 _ _]
          frame #0 {
            n407 = Empty String/Path?(string/path=w697) -> (empty?=w698:bool)
            n408 = case shown="False" w698 {
              tunnel: w697 -> [w719 _]
              tunnel: [w718 _] -> _
              tunnel: [w717 _] -> w700
              frame False {
                n409 = call <vilib>:"Read JPEG File.vi"("path to JPEG file"=w719) -> ("error out"=w718:errorcluster, "image data"=w717:T48)  [unwired: 8 in, 1 out]
              }
              frame True {
              }
            }
            n410 = call <vilib>:"Draw Flattened Pixmap.vi"("image data"=w700, "picture"=picture data[5B]) -> ("new picture"=w715:picture)  [unwired: 7 in]
            n411 = call <vilib>:"Picture to Pixmap.vi"("picture"=w715) -> ("image data"=w701:T48)  [unwired: 9 in, 1 out]
            n412 = Unbundle By Name(w701) -> ("image depth"=w712:i32, "Rectangle.right"=w710:i16, "Rectangle.left"=w709:i16, "Rectangle.bottom"=w708:i16, "Rectangle.top"=w707:i16)
            n413 = Compound Arithmetic op=ADD(w710, invert w709) -> (w706:i16)
            n414 = Compound Arithmetic op=ADD(w708, invert w707) -> (w705:i16)
            n415 = Bundle By Name(cluster=cluster{"Width":u32, "Height":u32} {"Width"=1000, "Height"=1000} ("Draw Area Size"), "Width"=w706, "Height"=w705) -> (w704:cluster{"Width":u32, "Height":u32})
            n416 = call "Picture Control to 2D Pixmap.vi"("Picture"=w715, "image depth"=w712, "Draw Area Size"=w704) -> ("24-bit"=w713:u32[][])  [unwired: 1 in, 3 out]
            n417 = call-poly "rotate pixmap.vi"("Rotation Angle (degrees)"=90.0, "Pixmap"=w713) -> ("Rotated Pixmap"=w714:u32[][])  [unwired: 2 in]
            n418 = call <vilib>:"Draw True-Color Pixmap(6_1).vi"("picture"=picture data[5B], "data (RGB format)"=w714) -> ("new picture"=w716:picture)  [unwired: 7 in]
            n419 = local write "Image"(w716) -> ()
            n420 = call "citTemplate.writeQueue.vi"("event in (if not connected:all statemachine with data event)"=ChangeOverGui.Action."Check" ("Action")) -> ()  [unwired: 14 in, 1 out]
          }
          frame #1 {
            n421 = Unbundle By Name(w720) -> ("WabcoPlate"=w723:string)
            n422 = Concatenate Strings(w723, ".png" ("string")) -> (w721:string)
            n423 = Build Path(base path=w726, name or relative path=w721) -> (appended path=w725:path)
            n424 = call "File exists.vi"("file path"=w725) -> ("exists?"=w727:bool)  [unwired: 4 in]
            n425 = case shown="True" w727 {
              tunnel: w725 -> [_ w732]
              tunnel: [_ w731] -> w729
              tunnel: [_ w730] -> _
              frame False {
              }
              frame True {
                n426 = call <vilib>:"Read PNG File.vi"("path to PNG file"=w732) -> ("error out"=w730:errorcluster, "image data"=w731:T48)  [unwired: 8 in, 1 out]
              }
            }
            n427 = call <vilib>:"Draw Flattened Pixmap.vi"("image data"=w729, "picture"=picture data[5B]) -> ("new picture"=w724:picture)  [unwired: 7 in]
            n428 = local write "WabcoPlate"(w724) -> ()
          }
          frame #2 {
            n429 = Unbundle By Name(w739) -> ("ClientPlate"=w735:string)
            n430 = Concatenate Strings(w735, ".png" ("string")) -> (w734:string)
            n431 = Build Path(base path=w738, name or relative path=w734) -> (appended path=w737:path)
            n432 = call "File exists.vi"("file path"=w737) -> ("exists?"=w740:bool)  [unwired: 4 in]
            n433 = case shown="True" w740 {
              tunnel: w737 -> [_ w745]
              tunnel: [_ w744] -> w742
              tunnel: [_ w743] -> _
              frame False {
              }
              frame True {
                n434 = call <vilib>:"Read PNG File.vi"("path to PNG file"=w745) -> ("error out"=w743:errorcluster, "image data"=w744:T48)  [unwired: 8 in, 1 out]
              }
            }
            n435 = call <vilib>:"Draw Flattened Pixmap.vi"("image data"=w742, "picture"=picture data[5B]) -> ("new picture"=w736:picture)  [unwired: 7 in]
            n436 = local write "ClientPlate"(w736) -> ()
          }
        }
      }
      frame "Check" {
        n437 = stacked-sequence {
          tunnel: w747 -> [w759 w777 w812]
          tunnel: w746 -> [_ _ _]
          frame #0 {
            n438 = Unbundle By Name(w759) -> ("WabcoProduct"=w756:string, "WabcoPlate"=w755:string, "ClientProduct"=w752:string, "ClientPlate"=w751:string, "TotalQuantity"=w758:u16, "OrderQuantity"=w749:u16, "Serial"=w750:i32)
            n439 = Bundle("WabcoProduct"=w756, "WabcoPlate"=w755) -> (w753:T49)  [unwired: 1 in]
            n440 = Bundle("ClientProduct"=w752, "ClientPlate"=w751) -> (w754:T50)  [unwired: 1 in]
            n441 = Bundle("TotalQuantity"=w758, "OrderQuantity"=w749, "Serial"=w750) -> (w757:T51)  [unwired: 1 in]
            n442 = local write "Wabco"(w753) -> ()
            n443 = local write "Client"(w754) -> ()
            n444 = local write "Serial"(w757) -> ()
          }
          frame #1 {
            n445 = Unbundle By Name(w777) -> ("WabcoPlate"=w764:string, "ClientPlate"=w778:string)
            n446 = call "ChangeOverGui.RefNumFormatStr.vi"("RefNum in"=w778) -> ("RefNum format ok?"=w762:bool)  [unwired: 2 out]
            n447 = call "ChangeOverGui.RefNumFormatStr.vi"("RefNum in"=w764) -> ("RefNum format ok?"=w763:bool)  [unwired: 2 out]
            n448 = property on="ShowPropertiesClient" class="Bool (strict)"() -> ("Value"=w773:bool)  [unwired: 2 in, 2 out]
            n449 = Compound Arithmetic op=AND(w763, w762) -> (w761:bool)
            "DoubleOrder" <- w761
            n450 = Compound Arithmetic op=AND(w761, w773) -> (w768:bool)
            n451 = property on="ShowPropertiesWabco" class="Bool (strict)"() -> ("Value"=w767:bool)  [unwired: 2 in, 2 out]
            n452 = Select(t=T15."Enabled" ("Disabled"), s=w761, f=T15."Disabled and Grayed Out" ("Disabled")) -> (s? t:f=w774:T15)
            n453 = property on="ShowPropertiesClient" class="Bool (strict)"("DisabledEnum"=w774, "Value"=w768) -> ()  [unwired: 2 in, 2 out]
            n454 = Compound Arithmetic op=OR(w768, w767) -> (w766:bool)
            n455 = Select(t=enum16{"-", "Wabco", "Client"}."Wabco" ("ViewMode"), s=w767, f=enum16{"-", "Wabco", "Client"}."-" ("ViewMode")) -> (s? t:f=w771:enum16{"-", "Wabco", "Client"})
            n456 = property on="Properties" class="Clust (strict)"("Visible"=w766) -> ()  [unwired: 2 in, 2 out]
            n457 = Select(t=enum16{"-", "Wabco", "Client"}."Client" ("ViewMode"), s=w768, f=w771) -> (s? t:f=w760:enum16{"-", "Wabco", "Client"})
            n458 = local write "ViewMode"(w760) -> ()
            n459 = property on="Progress" class="Bool (strict)"("Visible"=FALSE) -> ()  [unwired: 2 in, 2 out]
          }
          frame #2 {
            n460 = local read "ViewMode"() -> (w780:enum16{"-", "Wabco", "Client"})
            n461 = case shown="Default" w780 {
              tunnel: w812 -> [w814 w816]
              tunnel: [w813 w815] -> w811
              frame Default {
                n462 = Unbundle By Name(w814) -> ("Wabco"=w813:T5)
              }
              frame "Client" {
                n463 = Unbundle By Name(w816) -> ("Client"=w815:T5)
              }
            }
            n464 = global read "V7310.Global.vi" "Laser.Status"() -> (w796:T39)
            n465 = Unbundle By Name(w796) -> ("Jobs"=w797:string[])
            n466 = Unbundle By Name(w811) -> ("LaserJob"=w793:string, "AdditionalTxt"=w810:string, "FactoryCode"=w809:string, "RevID"=w808:u8, "ForkID"=w807:u8, "FailuresLimit"=w806:u16, "GlobalCnt"=w805:i32, "ScannerProgram"=w804:u8, "SerialFormat"=w803:T6, "CoordA"=w802:T7, "CoordB"=w801:T7, "CVX_Program"=w779:u16, "DMCconfig"=w788:i32)
            n467 = global read "Station.Global.vi" "DMCdata"() -> (w789:T44[])
            n468 = Build Array (concatenate)("", w797) -> (w795:string[])
            n469 = Index Array(array=w789, index=w788) -> (element=w787:T44)
            n470 = Search 1D Array(1D array=w795, element=w793) -> (index of element=w798:i32)  [unwired: 1 in]
            n471 = Unbundle By Name(w787) -> ("Name"=w786:string)
            n472 = Max & Min(x=w798, y=0) -> (max(x,y)=w792:i32)  [unwired: 1 out]
            n473 = Bundle By Name(cluster="Properties", "LaserJob"=w792, "AddTxt"=w810, "FactoryCode"=w809, "RevID"=w808, "ForkID"=w807, "Failures Limit"=w806, "GlobalCounter"=w805, "Bank"=w804, "SerialFormat"=w803, "CodeA"=w802, "CodeB"=w801, "CVX Program"=w779, "SetupDMC"=FALSE) -> (w800:T1)
            n474 = property on="LaserJob" class="Ring (strict)"("Strings []"=w795) -> ()  [unwired: 2 in, 2 out]
            n475 = String Subset(string=w786, length (rest)=15 ("length (rest)")) -> (substring=w782:string)  [unwired: 1 in]
            n476 = local write "Properties"(w800) -> ()
            n477 = call "Sequence.Test.DMC.GetDMCSize.vi"() -> ("max size"=w784:i32)  [unwired: 11 in]
            n478 = Format Into String(format string="%s #%d", w782, w784) -> (resulting string=w781:string)  [unwired: 2 in, 1 out]
            n479 = property on="SetupDMC" class="Bool (strict)"("BoolText.Text"=w781) -> ()  [unwired: 2 in, 2 out]
          }
        }
      }
      frame "Accept" {
        n480 = global write "Station.Global.vi" "+1 week"(FALSE ("+1 week")) -> ()
        n481 = call "citTemplate.writeQueue.vi"("event in (if not connected:all statemachine with data event)"=ChangeOverGui.Action."Clear" ("Action")) -> ()  [unwired: 14 in, 1 out]
        n482 = global read "Config.Global.vi" "IgnoreWabcoNoFormat"() -> (w819:bool)
        n483 = case shown="True" w819 {
          tunnel: Translator.Message."Formatting of WabcoNo is disabled. Do you want to continue?" ("_Msg") -> [_ w828]
          tunnel: [TRUE ("ok") w827] -> w817
          frame False {
          }
          frame True {
            n484 = call "InfoGui.vi"("_Msg"=w828) -> ("ok"=w827:bool)  [unwired: 10 in]
          }
        }
        n485 = case shown="True" w817 {
          tunnel: w825 -> [w829 w836]
          tunnel: [w829 w834] -> w824
          tunnel: w823 -> [w830 w833]
          tunnel: [w830 w831] -> w822
          frame False {
          }
          frame True {
            n486 = Bundle By Name(cluster=w833, "State"=Station.Changeover.State.vi."Ready" ("Changeover state")) -> (w831:T3)
            n487 = call "Logger.Variant.Write.vi"("error in (no error)"=w836, "VariantSets"=w831) -> ("error out"=w835:errorcluster)  [unwired: 9 in]
            n488 = call "Station-Order.vi"("error in (no error)"=w835, "VariantSets"=w831) -> ("error out"=w834:errorcluster)  [unwired: 9 in]
          }
        }
      }
      frame "Reject" {
        w837 = T3 {"State"=enum."Init", "ImgPath"=path "", "WabcoPlate"="", "WabcoProduct"="", "ClientProduct"="", "ClientPlate"="", "TotalQuantity"=0, "OrderQuantity"=0, "Serial"=0, "Wabco"={"LaserJob"="", "AdditionalTxt"="", "FactoryCode"="037", "RevID"=0, "ForkID"=0, "FailuresLimit"=0, "GlobalCnt"=0, "ScannerProgram"=0, "SerialFormat"=enum."6 dig", "CoordA"={"X"=0.0, "Y"=0.0, "Angle"=0.0}, "CoordB"={"X"=0.0, "Y"=0.0, "Angle"=0.0}, "DMCconfig"=0, "CVX_Program"=0}, "Client"={"LaserJob"="", "AdditionalTxt"="", "FactoryCode"="037", "RevID"=0, "ForkID"=0, "FailuresLimit"=0, "GlobalCnt"=0, "ScannerProgram"=0, "SerialFormat"=enum."6 dig", "CoordA"={"X"=0.0, "Y"=0.0, "Angle"=0.0}, "CoordB"={"X"=0.0, "Y"=0.0, "Angle"=0.0}, "DMCconfig"=0, "CVX_Program"=0}} ("t")
        n489 = global read "Sequence.Global.vi" "SeqData"() -> (w847:T30)
        n490 = Unbundle By Name(w847) -> ("Code.OrderDone"=w840:bool, "Code.Variant"=w839:T3)
        n491 = call "citTemplate.writeQueue.vi"("event in (if not connected:all statemachine with data event)"=ChangeOverGui.Action."Clear" ("Action")) -> ("error out"=w845:errorcluster)  [unwired: 14 in]
        n492 = Select(t=w837, s=w840, f=w839) -> ()  [unwired: 1 out]
        n493 = call "MainGui-ModeSelect.vi"("error in (no error)"=w842, "Mode"=Sequence.MainMode."Order" ("f")) -> ("error out"=w841:errorcluster)  [unwired: 9 in]
        n494 = call "citTemplate.writeQueue.vi"("event in (if not connected:all statemachine with data event)"=ChangeOverGui.Action."Read File" ("Action"), "error in (no error)"=w845) -> ()  [unwired: 13 in, 1 out]
        n495 = global write "Station.Global.vi" "+1 week"(FALSE ("+1 week")) -> ()
      }
      frame "Scan.Begin" {
        w854 = picture data[5B] ("picture")
        n496 = local write "Image"(w854) -> ()
        n497 = local write "WabcoPlate"(w854) -> ()
        n498 = local write "ClientPlate"(w854) -> ()
        n499 = call "citTemplate.writeQueue.vi"("event in (if not connected:all statemachine with data event)"=ChangeOverGui.Action."Clear" ("Action")) -> ("error out"=w848:errorcluster)  [unwired: 14 in]
        n500 = Bundle By Name(cluster=T3 {"State"=enum."Scaning", "ImgPath"=path "", "WabcoPlate"="", "WabcoProduct"="", "ClientProduct"="", "ClientPlate"="", "TotalQuantity"=0, "OrderQuantity"=0, "Serial"=0, "Wabco"={"LaserJob"="", "AdditionalTxt"="037", "FactoryCode"="", "RevID"=0, "ForkID"=0, "FailuresLimit"=0, "GlobalCnt"=0, "ScannerProgram"=0, "SerialFormat"=enum."6 dig", "CoordA"={"X"=0.0, "Y"=0.0, "Angle"=0.0}, "CoordB"={"X"=0.0, "Y"=0.0, "Angle"=0.0}, "DMCconfig"=0, "CVX_Program"=0}, "Client"={"LaserJob"="", "AdditionalTxt"="", "FactoryCode"="037", "RevID"=0, "ForkID"=0, "FailuresLimit"=0, "GlobalCnt"=0, "ScannerProgram"=0, "SerialFormat"=enum."6 dig", "CoordA"={"X"=0.0, "Y"=0.0, "Angle"=0.0}, "CoordB"={"X"=0.0, "Y"=0.0, "Angle"=0.0}, "DMCconfig"=0, "CVX_Program"=0}} ("VariantSets"), "State"=Station.Changeover.State.vi."Scaning") -> (w851:T3)
        n501 = call "citTemplate.writeQueue.vi"("event in (if not connected:all statemachine with data event)"=ChangeOverGui.Action."Scan" ("Action"), "error in (no error)"=w848) -> ()  [unwired: 13 in, 1 out]
      }
      frame "Scan" {
        n502 = for {
          N: 7 -> [_]
          shift-right: [w868] -> w861
          shift-left: w863 -> [w870]
          shift-right: [w873] -> w865
          shift-left: w866 -> [w871]
          shift-right: [w867] -> _
          shift-left: _ -> [w872]
          i -> [w869]
          stop <- w868 stop-if-true
          n503 = case shown="3" w869 {
            selector: w869 -> [w877 w899 w916 w935 w946 w971 _ _]
            tunnel: w871 -> [w890 w908 w923 w942 w958 w970 w982 w999]
            tunnel: [w889 w907 w919 w931 w957 w965 w982 w999] -> w873
            tunnel: [w879 w903 w918 w933 w949 w959 w981 w998] -> w868
            tunnel: [w888 w906 w922 w941 w954 w973 w980 w1000] -> w867
            tunnel: w872 -> [_ w902 w921 w938 w955 w964 w983 w1000]
            tunnel: w870 -> [w892 w910 w925 w944 w950 w972 w981 w998]
            frame 0 {
              w884 = u32 16744576 ("color(black)")
              n504 = call "Keyence.Main-Scan.vi"("get img (F)"=TRUE, "Idx"=1, "error in"=w892, "Bank"=w877) -> ("error out"=w881:errorcluster, "Code"=w891:T52)  [unwired: 5 in, 1 out]
              n505 = Unbundle By Name(w891) -> ("text"=w886:string, "corners"=w887:cluster{"X":i32, "Y":i32}[], "path"=w874:path)
              n506 = Empty String/Path?(string/path=w874) -> (empty?=w880:bool)
              n507 = call "ChangeOverGui.RefNumFormatStr.vi"("RefNum in"=w886) -> ("RefNum out"=w885:string)  [unwired: 2 out]
              n508 = case shown="False" w880 {
                tunnel: w881 -> [w897 w898]
                tunnel: w874 -> [w896 _]
                tunnel: [w895 w898] -> w879
                tunnel: [w894 _] -> w883
                frame False {
                  n509 = call <vilib>:"Read JPEG File.vi"("error in (no error)"=w897, "path to JPEG file"=w896) -> ("error out"=w895:errorcluster, "image data"=w894:T48)  [unwired: 7 in, 1 out]
                }
                frame True {
                }
              }
              n510 = Bundle By Name(cluster=w890, "State"=Station.Changeover.State.vi."NOK", "ImgPath"=w874, "WabcoProduct"=w885) -> (w889:T3)
              n511 = call <vilib>:"Draw Flattened Pixmap.vi"("image data"=w883, "picture"=picture data[5B]) -> ("new picture"=w878:picture)  [unwired: 7 in]
              n512 = call <vilib>:"Draw Multiple Lines.vi"("picture"=w878, "line endpoints"=w887, "color(black)"=w884) -> ("new picture"=w888:picture)  [unwired: 6 in]
              n513 = property on="ProductNo" class="Str"("Text.BGColor"=w884) -> ()  [unwired: 2 in, 2 out]
            }
            frame 1 {
              w900 = u32 16777088 ("color(black)")
              n514 = call "Keyence.Main-Scan.vi"("Idx"=1, "error in"=w910, "Bank"=w899) -> ("error out"=w903:errorcluster, "Code"=w909:T52)  [unwired: 6 in, 1 out]
              n515 = Unbundle By Name(w909) -> ("text"=w905:string, "corners"=w901:cluster{"X":i32, "Y":i32}[])
              n516 = call "ChangeOverGui.RefNumFormatStr.vi"("RefNum in"=w905) -> ("RefNum out"=w904:string)  [unwired: 2 out]
              n517 = Bundle By Name(cluster=w908, "WabcoPlate"=w904) -> (w907:T3)
              n518 = call <vilib>:"Draw Multiple Lines.vi"("picture"=w902, "line endpoints"=w901, "color(black)"=w900) -> ("new picture"=w906:picture)  [unwired: 6 in]
              n519 = property on="PlateNo" class="Str"("Text.BGColor"=w900) -> ()  [unwired: 2 in, 2 out]
            }
            frame 2 {
              w917 = u32 8454016 ("color(black)")
              n520 = call "Keyence.Main-Scan.vi"("Idx"=1, "error in"=w925, "Bank"=w916) -> ("error out"=w918:errorcluster, "Code"=w924:T52)  [unwired: 6 in, 1 out]
              n521 = Unbundle By Name(w924) -> ("text"=w914:string, "status"=w915:bool, "corners"=w920:cluster{"X":i32, "Y":i32}[])
              n522 = Select(t=w914, s=w915, f="") -> (s? t:f=w913:string)
              n523 = Bundle By Name(cluster=w923, "ClientProduct"=w913) -> (w919:T3)
              n524 = call <vilib>:"Draw Multiple Lines.vi"("picture"=w921, "line endpoints"=w920, "color(black)"=w917) -> ("new picture"=w922:picture)  [unwired: 6 in]
              n525 = property on="ProductNo" class="Str"("Text.BGColor"=w917) -> ()  [unwired: 2 in, 2 out]
            }
            frame 3 {
              w936 = u32 16744448 ("color(black)")
              n526 = call "Keyence.Main-Scan.vi"("Idx"=1, "error in"=w944, "Bank"=w935) -> ("error out"=w934:errorcluster, "Code"=w943:T52)  [unwired: 6 in, 1 out]
              n527 = Unbundle By Name(w943) -> ("text"=w940:string, "corners"=w937:cluster{"X":i32, "Y":i32}[])
              n528 = call "ChangeOverGui.RefNumFormatStr.vi"("RefNum in"=w940) -> ("RefNum out"=w939:string)  [unwired: 2 out]
              n529 = Bundle By Name(cluster=w942, "ClientPlate"=w939) -> (w932:T3)
              n530 = call "Logger.Variant.Read.vi"("error in (no error)"=w934, "VariantSets in"=w932) -> ("error out"=w933:errorcluster, "ClientPlateImg"=→"ClientPlate":picture, "WabcoPlateImg"=→"WabcoPlate":picture, "VariantSets out"=w931:T3, "OrdersTableIdx"=w927:i32, "OrdersTable"=w928:string[][])  [unwired: 4 in]
              n531 = property on="OrdersTable" class="MCListbox (strict)"("ItemNames"=w928, "Value"=w927) -> ()  [unwired: 2 in, 2 out]
              n532 = call <vilib>:"Draw Multiple Lines.vi"("picture"=w938, "line endpoints"=w937, "color(black)"=w936) -> ("new picture"=w941:picture)  [unwired: 6 in]
              n533 = property on="PlateNo" class="Str"("Text.BGColor"=w936) -> ()  [unwired: 2 in, 2 out]
            }
            frame 4 {
              w953 = u32 16744703 ("color(black)")
              n534 = call "Keyence.Main-Scan.vi"("Idx"=1, "error in"=w950, "Bank"=w946) -> ("error out"=w949:errorcluster, "Code"=w951:T52)  [unwired: 6 in, 1 out]
              n535 = Unbundle By Name(w951) -> ("text"=w948:string, "corners"=w947:cluster{"X":i32, "Y":i32}[])
              n536 = call "Str2Int.vi"("string"=w948) -> ("Numeric"=w956:i32)
              n537 = Bundle By Name(cluster=w958, "TotalQuantity"=w956) -> (w957:T3)
              n538 = call <vilib>:"Draw Multiple Lines.vi"("picture"=w955, "line endpoints"=w947, "color(black)"=w953) -> ("new picture"=w954:picture)  [unwired: 6 in]
              n539 = property on="TotalQuantity" class="DigNum (strict)"("NumText.BGColor"=w953) -> ()  [unwired: 2 in, 2 out]
            }
            frame 5 {
              w969 = u32 8454143 ("color(black)")
              n540 = call "Keyence.Main-Scan.vi"("Idx"=1, "error in"=w972, "Bank"=w971) -> ("error out"=w959:errorcluster, "Code"=w966:T52)  [unwired: 6 in, 1 out]
              n541 = Unbundle By Name(w966) -> ("text"=w961:string, "corners"=w967:cluster{"X":i32, "Y":i32}[])
              n542 = call <vilib>:"Trim Whitespace.vi"("string"=w961) -> ("trimmed string"=w960:string)  [unwired: 1 in]
              n543 = Decimal Digit?(1:w960) -> (0:w962:bool)
              n544 = case shown="True" w962 {
                tunnel: [w978 -1 ("Numeric")] -> w963
                tunnel: w960 -> [w974 _]
                frame True {
                  n545 = call <vilib>:"Space Constant.vi"() -> ("String"=w976:string)
                  n546 = Search and Replace String(replace all?=TRUE ("replace all? (F)"), input string=w974, search string=w976) -> (result string=w977:string)  [unwired: 5 in, 3 out]
                  n547 = call "Str2Int.vi"("string"=w977) -> ("Numeric"=w978:i32)
                }
                frame False {
                }
              }
              n548 = Bundle By Name(cluster=w970, "Serial"=w963) -> (w965:T3)
              n549 = call <vilib>:"Draw Multiple Lines.vi"("picture"=w964, "line endpoints"=w967, "color(black)"=w969) -> ("new picture"=w973:picture)  [unwired: 6 in]
              n550 = property on="SerialNo" class="DigNum (strict)"("NumText.BGColor"=w969) -> ()  [unwired: 2 in, 2 out]
            }
            frame 6 {
              n551 = call <vilib>:"Picture to Pixmap.vi"("picture"=w983) -> ("image data"=w984:T48)  [unwired: 9 in, 1 out]
              n552 = Unbundle By Name(w984) -> ("image depth"=w995:i32, "Rectangle.right"=w993:i16, "Rectangle.left"=w992:i16, "Rectangle.bottom"=w991:i16, "Rectangle.top"=w990:i16)
              n553 = Compound Arithmetic op=ADD(w993, invert w992) -> (w989:i16)
              n554 = Compound Arithmetic op=ADD(w991, invert w990) -> (w988:i16)
              n555 = Bundle By Name(cluster=cluster{"Width":u32, "Height":u32} {"Width"=1000, "Height"=1000} ("Draw Area Size"), "Width"=w989, "Height"=w988) -> (w987:cluster{"Width":u32, "Height":u32})
              n556 = call "Picture Control to 2D Pixmap.vi"("Picture"=w983, "image depth"=w995, "Draw Area Size"=w987) -> ("24-bit"=w996:u32[][])  [unwired: 1 in, 3 out]
              n557 = call-poly "rotate pixmap.vi"("Rotation Angle (degrees)"=90.0, "Pixmap"=w996) -> ("Rotated Pixmap"=w997:u32[][])  [unwired: 2 in]
              n558 = call <vilib>:"Draw True-Color Pixmap(6_1).vi"("picture"=picture data[5B], "data (RGB format)"=w997) -> ("new picture"=w980:picture)  [unwired: 7 in]
              "Image" <- w980
            }
            frame Default {
            }
          }
        }
        n559 = call "Keyence.Main-GetTablePosition.vi"("error in (no error)"=w863, "ScannerSlot in"=0) -> ("error out"=w860:errorcluster, "ScannerSlot out"=w862:i32)  [unwired: 7 in, 1 out]
        n560 = global write "Station.Global.vi" "ScannerSlot"(w862) -> ()
        n561 = Merge Errors(w861, w860) -> (w859:errorcluster)
        n562 = property on="Progress" class="Bool (strict)"("Visible"=TRUE) -> ()  [unwired: 2 in, 2 out]
        n563 = call "citTemplate.writeQueue.vi"("event in (if not connected:all statemachine with data event)"=ChangeOverGui.Action."Check" ("Action")) -> ()  [unwired: 14 in, 1 out]
      }
      frame "Update Table" {
        n564 = property on="OrdersTable" class="MCListbox (strict)"() -> ("ItemNames"=w1011:string[][], "Value"=w1004:i32, "TopLeft"=w1003:T12, "NumRows"=w1008:u32)  [unwired: 2 in, 2 out]
        n565 = Array Size(array=w1011) -> (size(s)=w1010:i32[])
        n566 = Unbundle By Name(w1003) -> ("Row"=w1016:u32)
        n567 = Index Array(array=w1010) -> (element=w1009:i32)  [unwired: 1 in]
        n568 = To Long Integer(number=w1016) -> (32bit integer=w1005:i32)
        n569 = To Long Integer(number=w1008) -> (32bit integer=w1006:i32)
        n570 = Compound Arithmetic op=ADD(invert 1 ("value"), w1005, w1006) -> (w1007:i32)
        n571 = In Range and Coerce(upper limit=w1007, x=w1004, lower limit=w1005) -> (coerced(x)=w1017:i32, In Range?=w1015:bool)
        n572 = Compound Arithmetic op=ADD(invert w1017, w1004, w1005) -> (w1014:i32)
        n573 = Select(t=w1005, s=w1015, f=w1014) -> (s? t:f=w1018:i32)
        n574 = In Range and Coerce(upper limit=w1009, x=w1018, lower limit=0) -> (coerced(x)=w1020:i32)  [unwired: 1 out]
        n575 = Bundle By Name(cluster=w1003, "Row"=w1020) -> (w1012:T12)
        n576 = property on="OrdersTable" class="MCListbox (strict)"("TopLeft"=w1012) -> ()  [unwired: 2 in, 2 out]
      }
      frame "Update Counter" {
        n577 = global read "Sequence.Global.vi" "SeqData"() -> (w1028:T30)
        n578 = Unbundle By Name(w1028) -> ("Code"=w1027:T37, "Code.Plate"=w1024:T11)
        n579 = To Word Integer(number=w1021) -> (16bit integer=w1026:i16)
        n580 = Decrement(x=w1026) -> (x-1=w1025:i16)
        n581 = To Word Integer(number=w1024) -> (16bit integer=w1023:i16)
        n582 = Equal?(x=w1023, y=w1025) -> (x = y?=w1022:bool)
        n583 = case shown="True" w1022 {
          tunnel: w1027 -> [_ w1035]
          frame False {
          }
          frame True {
            n584 = call "Sequence.PlateDetailsGet.vi"("Code in"=w1035) -> ("PlateDetails"=w1034:T5)  [unwired: 9 in, 1 out]
            n585 = Unbundle By Name(w1034) -> ("GlobalCnt"=w1031:i32)
            n586 = local read "Properties"() -> (w1033:T1)
            n587 = Bundle By Name(cluster=w1033, "GlobalCounter"=w1031) -> (w1032:T1)
            n588 = local write "Properties"(w1032) -> ()
          }
        }
      }
      frame "DMC Accept" {
        n589 = Unflatten From String(type=0, binary string=w1045, error in (no error)=w1044) -> (value=w1041:i32, error out=w1039:errorcluster)  [unwired: 3 out]
        n590 = case shown="\"Wabco\"" w1036 {
          tunnel: w1042 -> [w1047 w1050 w1053]
          tunnel: [w1047 w1049 w1052] -> w1037
          tunnel: w1041 -> [_ w1048 w1051]
          frame "-" {
          }
          frame "Wabco" {
            n591 = Bundle By Name(cluster=w1050, "Wabco.DMCconfig"=w1048) -> (w1049:T3)
          }
          frame "Client" {
            n592 = Bundle By Name(cluster=w1053, "Client.DMCconfig"=w1051) -> (w1052:T3)
          }
        }
        n593 = call "Logger.Variant.Write.vi"("error in (no error)"=w1039, "VariantSets"=w1037) -> ("error out"=w1038:errorcluster)  [unwired: 9 in]
        n594 = call "citTemplate.writeQueue.vi"("event in (if not connected:all statemachine with data event)"=ChangeOverGui.Action."Check" ("Action")) -> ()  [unwired: 14 in, 1 out]
      }
    }
    n595 = Unbundle By Name(w2) -> ("State"=w4:T4)
    n596 = global write "Station.Global.vi" "OrderSets"(w2) -> ()
    n597 = call "citTemplate.sendAckNotifier.vi"("notification data"=w14, "notifierHandle in"=w15, "error in"=w12) -> ()  [unwired: 13 out]
    n598 = global write "Station.Global.vi" "Changeover state"(w4) -> ()
    n599 = call "citTemplate.ErrorEventPass.vi"("error in"=w12, "action of error"=w8, "event in"=w13) -> ("error out"=w7:errorcluster)  [unwired: 2 in, 6 out]
  }
